vi "CH_LM Getting Started.vi"(5 "ID Query? (T: Yes)":bool, 7 "Reset? (F: No)":bool) -> ()   [LabVIEW 2012, in "CH_LM.lvlib"]
doc: "This example VI can be used to test the communication with a connected LabMax device and a connected detector.\n\n<B>Hint:</B> The control on the rigt side are immediatly updated with values read from the device. So, if value does not change and no error occurred you request was executed sucessfully."
uses:
  CH_LM.lvlib
  <vilib>/Utility/error.llb/DialogType.ctl
  Instance           1 29Saved   CH_LM Getting Started .vi
  CH_LM Measurement Mode.ctl
  CH_LM Unit.ctl
  CH_LM Measurement Delivery Mode.ctl
  CH_LM Date Format.ctl
  CH_LM Meter Type.ctl
  CH_LM ProbeType.ctl
  CH_LM AnalogOutFullscaleVoltage.ctl
  CH_LM Numeric Resolution.ctl
  CH_LM Time.ctl
  CH_LM Statistics Display Item.ctl
  CH_LM Display Mode.ctl
  CH_LM Display Submode.ctl
  CH_LM View Mode.ctl
  CH_LM Trigger Bus Control.ctl
  CH_LM Trigger Source.ctl
  CH_LM Zoom Factor.ctl
  CH_LM File Information.ctl
  CH_LM Data Token.ctl
  CH_LM Streaming Data.ctl
  CH_LM System StatusCluster.ctl
  CH_LM ProbeQualifier.ctl
  CH_LM BaudRates.ctl
  CH_LM Parity.ctl
  CH_LM SerialConfiguration.ctl
panel:
  in  "stop":bool
  in  "Unlock? (True)":bool
  out "GUI Loop":i32
  out "stopping":bool
  out "SRQ error":bool
  out "SRQ":bool
  out "Polling error":bool
  out "Streaming error":bool
  out "Lock timed out":bool
  in  "Reset 4":bool
  out "Event error":errorcluster
  in  "Tab Control":T1(tab)
  out "Probe Diameter":dbl[unit] format="%#.2g"
  out "Probe Qualifier":T2
  in  "Update Probe":bool
  out "Responsitivity":dbl format="%#.1g"
  out "Calibration Date":timestamp format="%<%x>T"
  out "Serial Number":string
  out "Probe Type":T3
  out "Probe Model":string
  out "Meter Type":T4
  out "Serial Number":string
  out "Calibration Date":string
  out "Self-Test Result Message":string
  out "Self-Test Result Code":i32
  out "Lock timed out":bool
  out "Date":string
  out "Revision":string
  out "Instrument Driver Revision":string
  out "Vendor":string
  out "Module":string
  out "timed out?":bool
  in  "Address":i32=1
  in  "Serial Number":string
  in  "Serial Configuration\n(19200,N,8,1)":T5={"Baud Rate"=19200, "Parity"=0, "Data Bits"=8, "Stop Bits"=1} {"Parity" items=["None", "Odd", "Even"]; "Baud Rate" items=["9600"=9600, "19200"=19200, "38400"=38400, "57600"=57600, "115200"=115200]}
  in  "Pyroelectric Autoset":bool
  out "Zero Offset / W":dbl format="%#.3g"
  in  "Probe zero":bool
  in  "Reset":bool
  out "Number of files":i32
  out "Configuration Catalog":string[](array[string])
  in  "Delete":bool
  in  "Save":bool
  in  "Recall":bool
  in  "Rename":bool
  in  "Destination File Name (\"\")":string
  in  "Source File Name (\"\")":string
  in  "Update Catalog":bool
  in  "Range Option (Value)":enum16{"MINIMUM", "Value", "MAXIMUM"}(ring)=enum."Value"
  in  "Range":dbl=1.0
  in  "Auto Range (disable)":bool
  in  "Analog Out Fullscale Voltage (2V)":T8=enum."2 V"
  in  "Time / s (0:Auto)":i32
  in  "Number of Pulses (0:Auto)":i32
  in  "Aperture / cm² (1.0)":dbl=1.0 format="%#.2g"
  in  "Area Correction (disable)":bool
  in  "Compensation Factor (1.0)":dbl=1.0 format="%#.3g"
  in  "Gain Compensation (disable)":bool
  in  "Resolution (3 1/2)":T9
  in  "Speedup Status":T10
  in  "set Measurement Mode":bool
  in  "Unit":T11
  in  "Mode":T12
  in  "State (On)":bool=TRUE
  in  "Battery Auto Off Timer (1 min)":i32=1
  in  "Battery Auto Off (On)":bool
  in  "AC Auto Off Timer (1 min)":i32=1
  in  "AC Auto Off (On)":bool
  in  "Date Format (MDY)":T13
  in  "Time Stamp":timestamp format="%<%X\n%x>T"
  in  "Factor (1)":T14=enum."1"
  in  "Direction (horizontal)":bool
  in  "Display Mode":bool
  in  "Tune Clear":bool
  in  "Clear (false)":bool
  in  "Text (empty)":string
  in  "Contrast (0.5)":dbl=0.5 min=0.0 max=1.0 step=0.1 format="%#_3g"
  in  "Set Display Mode":bool
  in  "View Mode":T15
  in  "Display Submode":T16
  in  "Display Mode":T17
  in  "Sequence ID (0)":u32
  in  "Trigger Source":T18
  in  "Release":bool
  in  "Hold":bool
  in  "Trigger Bus Control (2)":T19=enum."Independent"
  in  "Trigger Delay (0µs)":dbl=5.0 format="%#.3g"
  in  "Trigger Slope (pos.)":bool=TRUE
  in  "Trigger Level (5%)":dbl=5.0 format="%#.3g"
  out "size":i32
  in  "set WL Table":bool
  in  "Wavelength Table":u32[](array[numeric])
  in  "WL correction (disable)":bool=TRUE
  in  "set Wavelength":bool
  in  "Option (Value)":enum16{"MINIMUM", "Value", "MAXIMUM"}(ring)=enum."Value"
  in  "Wavelength / nm":u32=123
  in  "Display Item List":T20[](array[typedef])=[enum."Mean"]
  in  "Sample Rate /Hz (10Hz)":dbl=10.0 format="%#.3e"
  in  "Sample Rate (1)":i32=1
  in  "Batch Time (00:01:00)":T21={"Hours"=0, "Minutes"=1, "Seconds"=0}
  in  "Batch Size (2)":i32=2
  in  "Number of Bins (7)":i32=7
  in  "Restart Mode (f:manual)":bool=TRUE
  in  "Polling active":bool
  out "Head Temperature":dbl[unit](slide)=273.15 scale=263.15..373.15
  in  "Intervall / ms":u32=500
  out "Status":T22
  out "Status Description":string
  in  "Reset 2":bool
  out "Polling error":errorcluster
  in  "send SCPI":bool
  out "Response":string
  in  "NofStrings (-1:all)":i32=-1
  in  "SCPI Command/Query":string
  out "Response Array":string[](array[string])
  in  "Wait for SRQ active":bool
  out "Data String":string
  out "System Status":u32 format="%.0x"
  out "Status":T23
  out "Description":string
  out "SRQ error":errorcluster
  in  "Streaming active":bool
  out "Unit":string
  in  "Reset 3":bool
  out "Stream error":errorcluster
  in  "Delivery Mode":T24
  out "Steaming Data Chart":cluster{"Value":sgl, u32}[](graph)
  in  "Batch (start)":bool
  in  "Header (disable)":bool
  in  "Data Tokens":T25[](array[typedef])=[enum."Raw data"]
  out "Steaming Data Cluster":T26 {"Flags" format="%.0b"; "Unit ID" format="%.0b"; "Quad Distance"."Y" format="%#.1f"; "Quad Distance"."X" format="%#.1f"; "Value" format="%#.7e"}
  in  "Start/Stop (start)":bool=TRUE
  in  "Cycle Time (00:01:00)":T21={"Hours"=0, "Minutes"=1, "Seconds"=0}
  in  "File Name (\"\")":string
  in  "Sample Rate /Hz (10Hz) 2":dbl=10.0 format="%#.3e"
  in  "Trend Time (00:01:00)":T21={"Hours"=0, "Minutes"=1, "Seconds"=0}
  in  "Sampling Rate (1)":i32=1
  in  "Trend Size (2)":i32=2
  in  "Trend Histogram Bins (7)":i32=7
  in  "Trend Zoom (1)":T14=enum."1"
  in  "Trend Cycle (start)":bool=TRUE
  out "Current working directoy":string
  in  "Root":enum16{"\\loc", "\\usb"}(ring)
  in  "Destination (empty path)":path
  in  "Download":bool
  in  "Load from File":bool
  in  "Store into File":bool
  out "Catalog size":i32
  in  "Change Directory":bool
  in  "Create Directory":bool
  in  "Copy File":bool
  in  "Destination Name (\"\")":string
  in  "Rename":bool
  in  "Type":bool
  out "File":T27
  in  "Catalog index":u32
  in  "Delete File":bool
  out "Catalog":T27[](array[typedef])
  out "Bytes available":i32
  out "Bytes in use":i32
  in  "Read Catalog":bool
  # "Bus"
  # "External"
  # "Internal"
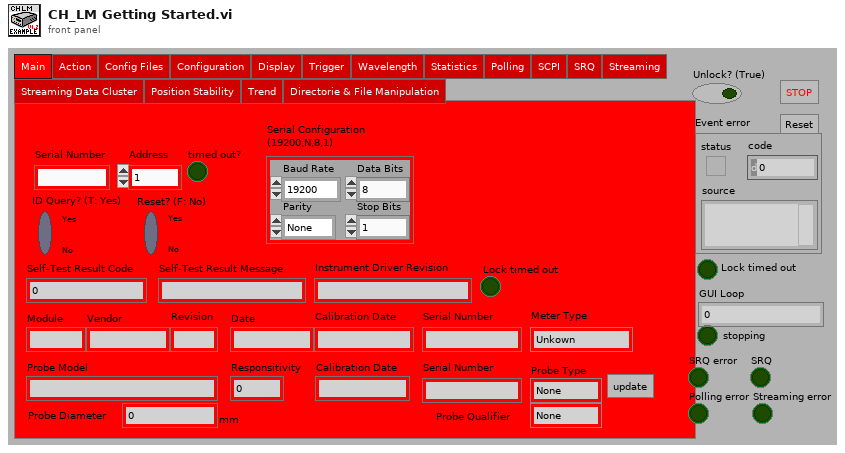
[diagram p1: front panel]
types:
  T1 = enum32{"Main", "Action", "Config Files", "Configuration", "Display", "Trigger", "Wavelength", "Statistics", "Polling", "SCPI", "SRQ", "Streaming", "Streaming Data Cluster", "Position Stability", "Trend", "Directorie & File Manipulation"}
  T2 = typedef "CH_LM.lvlib/CH_LM ProbeQualifier.ctl" = enum16{"None", "Single", "Quad", "No Spec"}
  T3 = typedef "CH_LM.lvlib/CH_LM ProbeType.ctl" = enum16{"None", "Thermopile", "Pyroelectric", "Optical"}
  T4 = typedef "CH_LM.lvlib/CH_LM Meter Type.ctl" = enum16{"Unkown", "TOP", "TO"}
  T5 = typedef "CH_LM.lvlib/CH_LM SerialConfiguration.ctl" = cluster{"Baud Rate":T6, "Parity":T7, "Data Bits":u16, "Stop Bits":u16}
  T6 = typedef "CH_LM.lvlib/CH_LM BaudRates.ctl" = u32
  T7 = typedef "CH_LM.lvlib/CH_LM Parity.ctl" = u16
  T8 = typedef "CH_LM.lvlib/CH_LM AnalogOutFullscaleVoltage.ctl" = enum16{"1 V", "2 V", "4 V"}
  T9 = typedef "CH_LM.lvlib/CH_LM Numeric Resolution.ctl" = enum16{"3½", "4½", "5½", "6½"}
  T10 = cluster{"Host":bool, "Analog":bool, "Numeric":bool, "Tune":bool}
  T11 = typedef "CH_LM.lvlib/CH_LM Unit.ctl" = enum16{"Joule", "Watt", "dBm"}
  T12 = typedef "CH_LM.lvlib/CH_LM Measurement Mode.ctl" = enum16{"Energy", "Power"}
  T13 = typedef "CH_LM.lvlib/CH_LM Date Format.ctl" = enum16{"MDY", "DMY"}
  T14 = typedef "CH_LM.lvlib/CH_LM Zoom Factor.ctl" = enum16{"Auto", "1", "2", "5", "10", "20"}
  T15 = typedef "CH_LM.lvlib/CH_LM View Mode.ctl" = enum16{"Scroll", "Fit to Screen", "Strip Chart", "Bar Chart"}
  T16 = typedef "CH_LM.lvlib/CH_LM Display Submode.ctl" = enum16{"Numbers", "Histogram", "Chart"}
  T17 = typedef "CH_LM.lvlib/CH_LM Display Mode.ctl" = enum16{"Non-Statistics", "Statistics", "Position Stability", "Tune", "Trend"}
  T18 = typedef "CH_LM.lvlib/CH_LM Trigger Source.ctl" = enum16{"Internal", "External", "Bus"}
  T19 = typedef "CH_LM.lvlib/CH_LM Trigger Bus Control.ctl" = enum16{"Host", "Guest", "Independent"}
  T20 = typedef "CH_LM.lvlib/CH_LM Statistics Display Item.ctl" = enum16{"Mean", "Minimum", "Maximum", "Standard Deviation", "1 Sigma", "2 Sigma", "3 Sigma", "Range", "Dose", "Missed"}
  T21 = typedef "CH_LM.lvlib/CH_LM Time.ctl" = cluster{"Hours":i32, "Minutes":i32, "Seconds":i32}
  T22 = cluster{"Battery":bool, "Temp":bool, "Probe":bool, "Drive":bool, "Autoset":bool, "Batch":bool, "Trend":bool, "Power":bool, "Trigger":bool, "Flash":bool, "FIFO":bool}
  T23 = typedef "CH_LM.lvlib/CH_LM System StatusCluster.ctl" = cluster{"Battery":bool, "Temp":bool, "Probe":bool, "Drive":bool, "Autoset":bool, "Batch":bool, "Trend":bool, "Power":bool, "Trigger":bool, "Flash":bool, "FIFO":bool, "Remote":bool, "Copy":bool}
  T24 = typedef "CH_LM.lvlib/CH_LM Measurement Delivery Mode.ctl" = enum16{"Last", "Stream"}
  T25 = typedef "CH_LM.lvlib/CH_LM Data Token.ctl" = enum16{"Raw data", "Quad distance", "Formated data", "Unit", "Pulse period", "Flags", "Sequence ID"}
  T26 = typedef "CH_LM.lvlib/CH_LM Streaming Data.ctl" = cluster{"Value":sgl, "Quad Distance":cluster{"X":sgl, "Y":sgl}, "Display Data":cluster{"Format ID":u8, "Scale ID":u8}, "Unit ID":u8, "Flags":u32, "Pulse Period":u32, "Sequence ID":u32, "Unit String":string}
  T27 = typedef "CH_LM.lvlib/CH_LM File Information.ctl" = cluster{"File name":string, "File type":string, "File size":i32}
  T28 = typedef "CH_LM.lvlib/CH_LM System Status.ctl" = u32
  T29 = cluster{"[0]":bool, "[1]":bool, "[2]":bool, "[3]":bool}
  T30 = cluster{"[0]":bool, "[1]":bool, "[2]":bool, "[3]":bool, "[4]":bool, "[5]":bool, "[6]":bool, "[7]":bool, "[8]":bool, "[9]":bool, "[10]":bool}
  T31 = typedef "DialogType.ctl" = u16
  T32 = typedef "CH_LM.lvlib/CH_LM Communication Mode.ctl" = enum16{"None", "USB", "GPIB", "RS232"}
  T33 = typedef "CH_LM File Information.ctl" = cluster{"File name":string, "File type":string, "File size":i32}
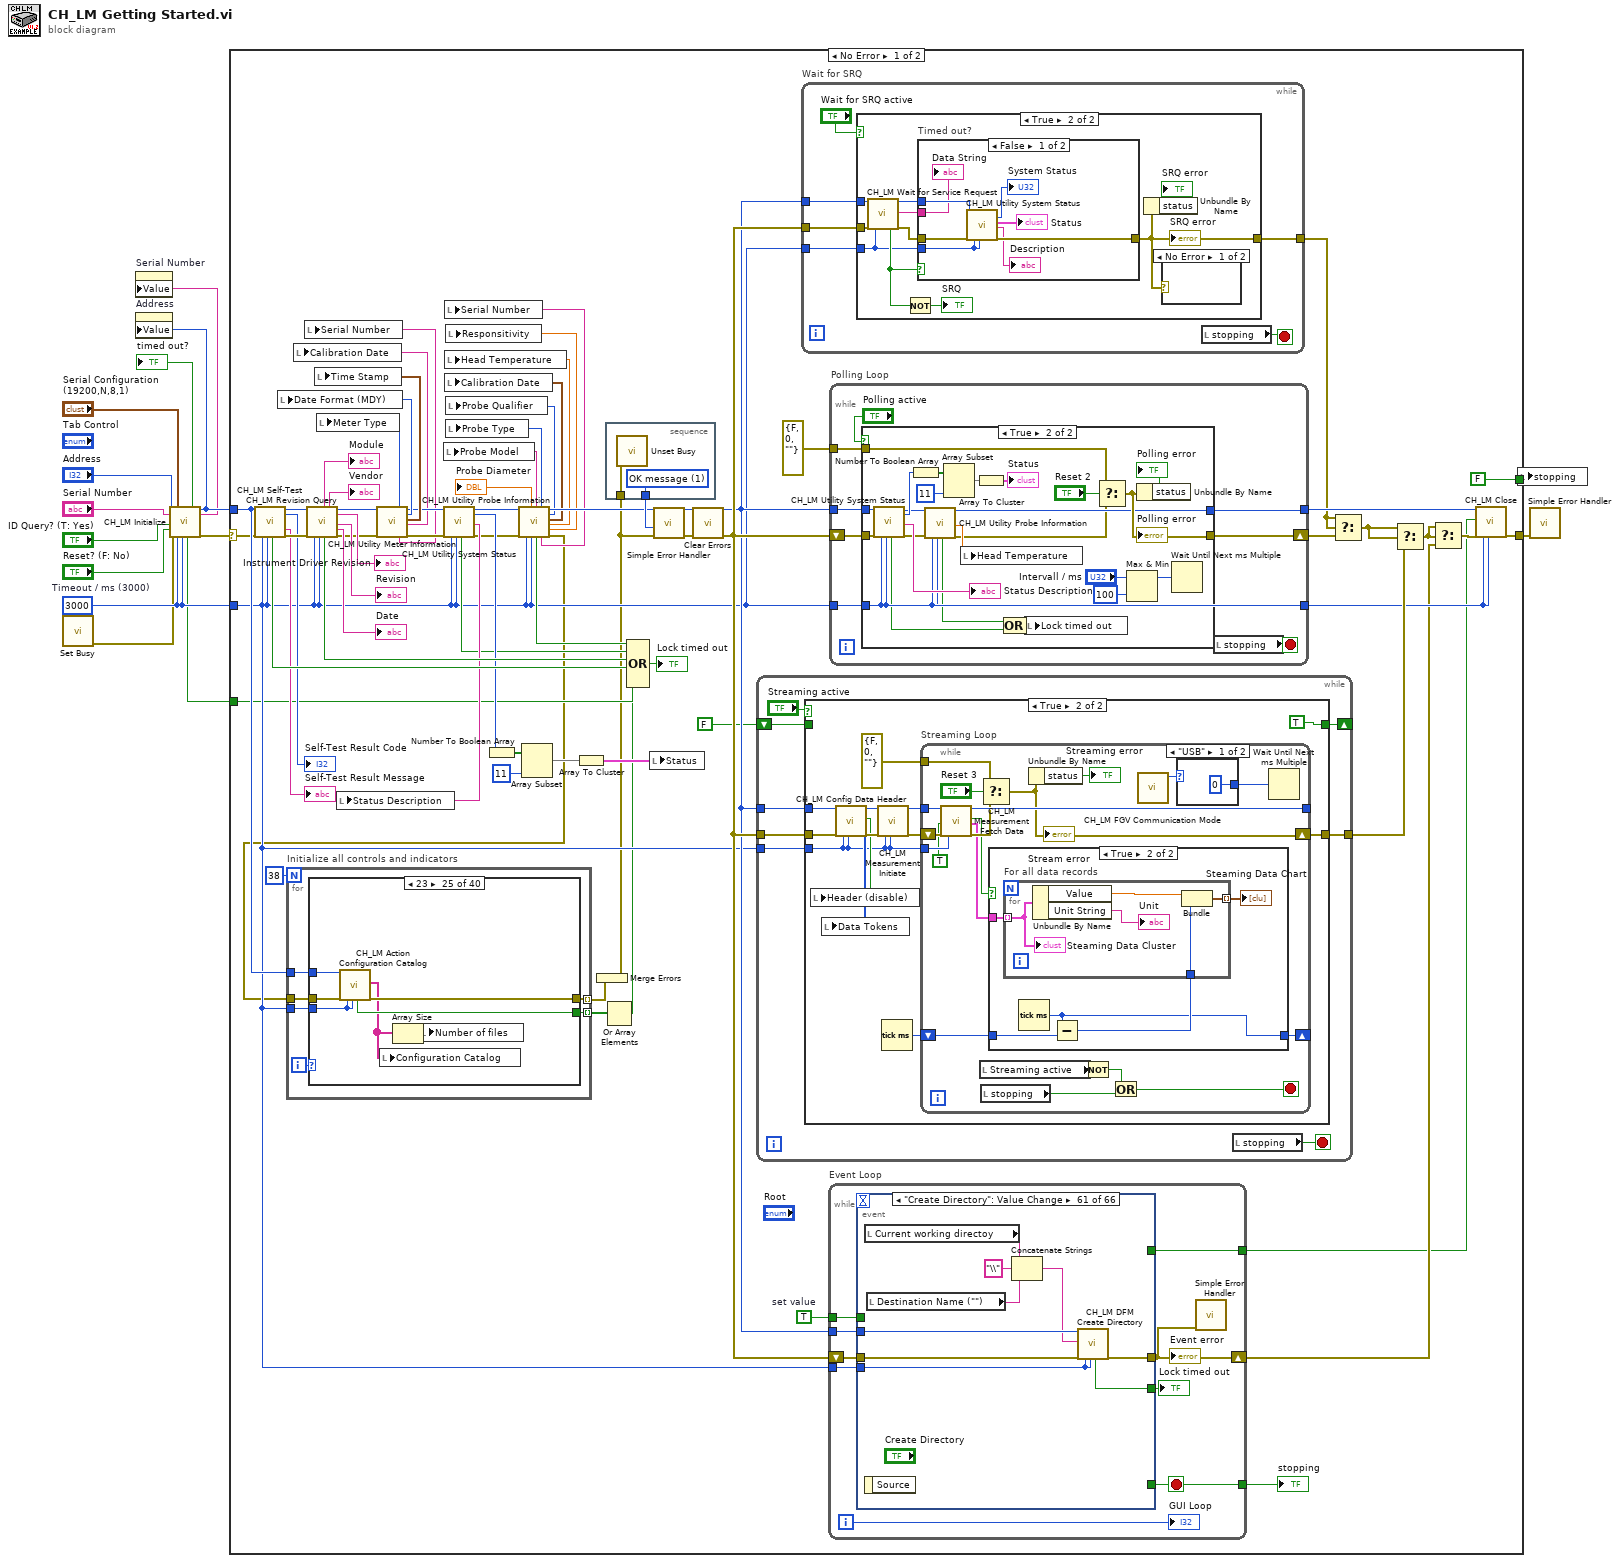
[diagram p0: block diagram]
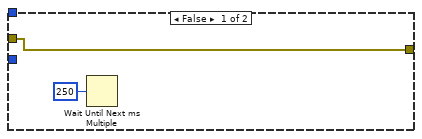
[diagram p2: hidden frame]
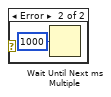
[diagram p3: hidden frame]
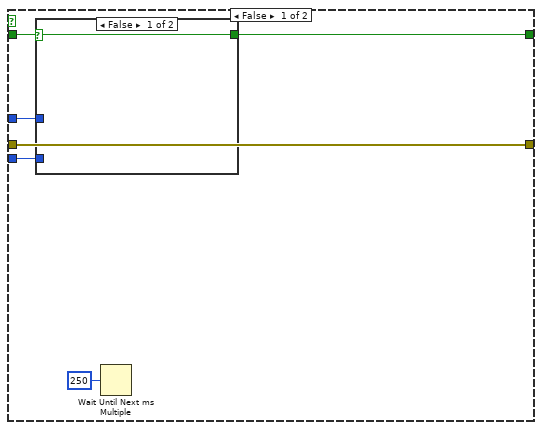
[diagram p5: hidden frame]
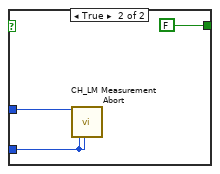
[diagram p6: hidden frame]
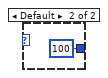
[diagram p7: hidden frame]
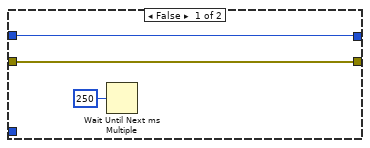
[diagram p9: hidden frame]
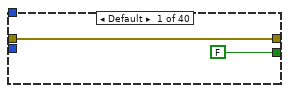
[diagram p10: hidden frame]
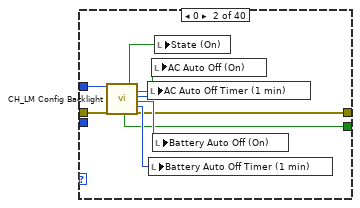
[diagram p11: hidden frame]
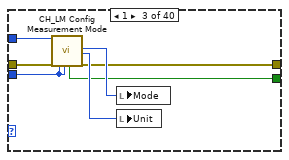
[diagram p12: hidden frame]
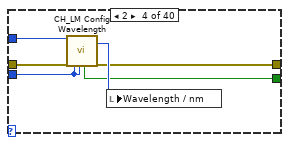
[diagram p13: hidden frame]
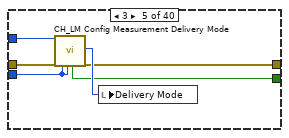
[diagram p14: hidden frame]
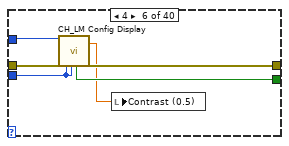
[diagram p15: hidden frame]
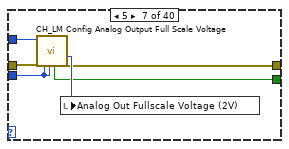
[diagram p16: hidden frame]
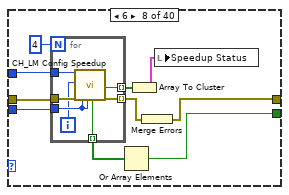
[diagram p17: hidden frame]
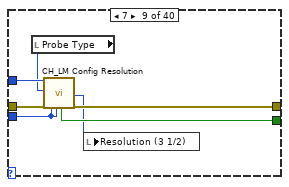
[diagram p18: hidden frame]
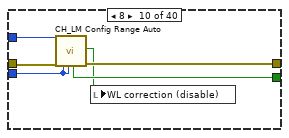
[diagram p19: hidden frame]
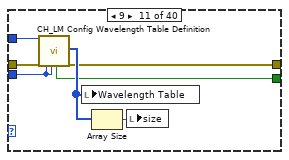
[diagram p20: hidden frame]
diagram:
  w11 = 3000  # Timeout / ms (3000)
  n1 = call <vilib>:"Set Busy.vi"() -> ("error out"=w4:errorcluster)  [unwired: 4 in, 7 out]
  n2 = call "CH_LM Initialize.vi"("Address"="Address", "Serial Number"="Serial Number", "ID Query (True)"="ID Query? (T: Yes)", "Reset (False)"="Reset? (F: No)", "error in (no error)"=w4, "Serial Configuration\n(19200,N,8,1)"="Serial Configuration\n(19200,N,8,1)", "Timeout / ms (3000)"=w11, "Lock Timeout / ms (1000)"=w11) -> ("Lock timed out"=w10:bool, "timed out?"=→"timed out?":bool, "Meter Index"=w3:i32, "Serial Number"=w2:string, "error out"=w8:errorcluster)  [unwired: 7 out]
  n3 = property on="Serial Number" class="Str"("Value"=w2) -> ()  [unwired: 2 in, 2 out]
  n4 = property on="Address" class="DigNum (strict)"("Value"=w3) -> ()  [unwired: 2 in, 2 out]
  n5 = case shown="No Error" w8 {
    selector: w8 -> [w28 w1239]
    tunnel: [w83 w1239] -> w14
    tunnel: w3 -> [w29 _]
    tunnel: w11 -> [w27 _]
    tunnel: w10 -> [w25 _]
    tunnel: [FALSE _] -> w7
    frame No Error {
      w64 = TRUE  # set value
      n6 = call "CH_LM Self-Test.vi"("Meter Index"=w29, "error in (no error)"=w28, "Timeout / ms (3000)"=w27, "Lock Timeout / ms (1000)"=w27) -> ("Lock timed out"=w70:bool, "Meter Index"=w74:i32, "Self-Test Result Code"=→"Self-Test Result Code":i32, "Self-Test Result Message"=→"Self-Test Result Message":string, "error out"=w73:errorcluster)  [unwired: 11 out]
      n7 = call "CH_LM Revision Query.vi"("Meter Index"=w74, "error in (no error)"=w73, "Timeout / ms (3000)"=w27, "Lock Timeout / ms (1000)"=w27) -> ("Module"=→"Module":string, "Lock timed out"=w71:bool, "Vendor"=→"Vendor":string, "Meter Index"=w47:i32, "Instrument Driver Revision"=→"Instrument Driver Revision":string, "Instrument Firmware Revision"=→"Revision":string, "Instrument Firmware Date"=→"Date":string, "error out"=w46:errorcluster)  [unwired: 8 out]
      n8 = call "CH_LM Utility Meter Information.vi"("Meter Index"=w47, "error in (no error)"=w46) -> ("Meter Type"=w44:T4, "Serial Number"=w42:string, "Meter Index"=w48:i32, "Date Format"=w51:T13, "Time Stamp"=w50:timestamp, "Calibration Date"=w43:string, "error out"=w45:errorcluster)  [unwired: 3 in, 8 out]
      n9 = local write "Date Format (MDY)"(w51) -> ()
      n10 = local write "Calibration Date"(w43) -> ()
      n11 = local write "Serial Number"(w42) -> ()
      n12 = local write "Time Stamp"(w50) -> ()
      n13 = local write "Meter Type"(w44) -> ()
      n14 = call "CH_LM Utility System Status.vi"("Meter Index"=w48, "error in (no error)"=w45, "Timeout / ms (3000)"=w27, "Lock Timeout / ms (1000)"=w27) -> ("Lock timed out"=w49:bool, "Meter Index"=w36:i32, "System Status"=w54:T28, "Status Description"=w52:string, "error out"=w37:errorcluster)  [unwired: 11 out]
      n15 = local write "Status Description"(w52) -> ()
      n16 = Number To Boolean Array(number=w54) -> (Boolean array=w56:bool[])
      n17 = call "CH_LM Utility Probe Information.vi"("Meter Index"=w36, "error in (no error)"=w37, "Timeout / ms (3000)"=w27, "Lock Timeout / ms (1000)"=w27) -> ("Probe Diameter"=→"Probe Diameter":dbl[unit], "Model"=w33:string, "Lock timed out"=w35:bool, "Probe Type"=w19:T3, "Serial Number"=w30:string, "Meter Index"=w34:i32, "Probe Qualifier"=w16:T2, "Calibration Date"=w32:timestamp, "Head Temperature"=w31:dbl[unit], "Responsitivity"=w17:dbl, "error out"=w22:errorcluster)  [unwired: 5 out]
      n18 = for "Initialize all controls and indicators" {
        N: 38 -> [_]
        tunnel: w29 -> [w217]
        tunnel: w22 -> [w213]
        tunnel: [w216] -> w23 mode=indexing
        tunnel: [w215] -> w26 mode=indexing
        tunnel: w27 -> [w214]
        i -> [w218]
        n19 = case shown="23" w218 {
          tunnel: w217 -> [_ w224 w234 w241 w247 w254 w259 w264 w284 w290 w296 w302 w308 w315 w321 w327 w332 w338 w344 w350 w356 w364 w370 w376 w386 w391 w397 w403 w409 w416 w422 w429 w437 w443 w449 w455 w462 w470 w480 w486]
          tunnel: w213 -> [w220 w223 w233 w240 w246 w253 w258 w266 w283 w289 w295 w301 w306 w314 w320 w326 w331 w337 w343 w349 w355 w363 w369 w375 w385 w389 w396 w402 w408 w415 w421 w428 w436 w442 w448 w454 w461 w469 w481 w485]
          tunnel: [w220 w222 w232 w237 w243 w250 w255 w263 w280 w286 w292 w298 w305 w311 w318 w323 w328 w334 w340 w347 w353 w360 w366 w372 w382 w388 w393 w399 w405 w412 w418 w425 w433 w440 w445 w451 w458 w466 w477 w482] -> w216
          tunnel: [FALSE ("Lock timed out") w221 w231 w238 w244 w251 w256 w267 w281 w287 w293 w299 w304 w312 w317 w324 w329 w335 w341 w346 w352 w361 w367 w373 w383 w387 w394 w400 w406 w413 w419 w426 w434 w439 w446 w452 w459 w467 w478 w483] -> w215
          tunnel: w214 -> [_ _ w230 w239 w245 w252 w257 w265 w282 w288 w294 w300 w307 w313 w319 w325 w330 w336 w342 w348 w354 w362 w368 w374 w384 w390 w395 w401 w407 w414 w420 w427 w435 w441 w447 w453 w460 w468 w479 w484]
          frame Default {
          }
          frame 0 {
            n20 = call "CH_LM Config Backlight.vi"("Meter Index"=w224, "error in (no error)"=w223) -> ("Lock timed out"=w221:bool, "State"=w225:bool, "AC Auto Off"=w226:bool, "AC Auto Off Timer / min"=w227:i32, "Battery Auto Off"=w228:bool, "Battery Auto Off Timer / min"=w229:i32, "error out"=w222:errorcluster)  [unwired: 6 in, 5 out]
            n21 = local write "AC Auto Off Timer (1 min)"(w227) -> ()
            n22 = local write "Battery Auto Off Timer (1 min)"(w229) -> ()
            n23 = local write "AC Auto Off (On)"(w226) -> ()
            n24 = local write "Battery Auto Off (On)"(w228) -> ()
            n25 = local write "State (On)"(w225) -> ()
          }
          frame 1 {
            n26 = call "CH_LM Config Measurement Mode.vi"("Meter Index"=w234, "error in (no error)"=w233, "Timeout / ms (3000)"=w230, "Lock Timeout / ms (1000)"=w230) -> ("Lock timed out"=w231:bool, "Mode"=w235:T12, "Unit"=w236:T11, "error out"=w232:errorcluster)  [unwired: 3 in, 9 out]
            n27 = local write "Mode"(w235) -> ()
            n28 = local write "Unit"(w236) -> ()
          }
          frame 2 {
            n29 = call "CH_LM Config Wavelength.vi"("Meter Index"=w241, "error in (no error)"=w240, "Timeout / ms (3000)"=w239, "Lock Timeout / ms (1000)"=w239) -> ("Lock timed out"=w238:bool, "Wavelength / nm"=w242:u32, "error out"=w237:errorcluster)  [unwired: 3 in, 10 out]
            n30 = local write "Wavelength / nm"(w242) -> ()
          }
          frame 3 {
            n31 = call "CH_LM Config Measurement Delivery Mode.vi"("Meter Index"=w247, "error in (no error)"=w246, "Timeout / ms (3000)"=w245, "Lock Timeout / ms (1000)"=w245) -> ("Lock timed out"=w244:bool, "Delivery Mode"=w248:T24, "error out"=w243:errorcluster)  [unwired: 2 in, 11 out]
            n32 = local write "Delivery Mode"(w248) -> ()
          }
          frame 4 {
            n33 = call "CH_LM Config Display.vi"("Meter Index"=w254, "error in (no error)"=w253, "Timeout / ms (3000)"=w252, "Lock Timeout / ms (1000)"=w252) -> ("Lock timed out"=w251:bool, "Contrast"=w249:dbl, "error out"=w250:errorcluster)  [unwired: 4 in, 9 out]
            n34 = local write "Contrast (0.5)"(w249) -> ()
          }
          frame 5 {
            n35 = call "CH_LM Config Analog Output Full Scale Voltage.vi"("Meter Index"=w259, "error in (no error)"=w258, "Timeout / ms (3000)"=w257, "Lock Timeout / ms (1000)"=w257) -> ("Lock timed out"=w256:bool, "Analog Out \nFullscale Voltage"=w260:T8, "error out"=w255:errorcluster)  [unwired: 2 in, 11 out]
            n36 = local write "Analog Out Fullscale Voltage (2V)"(w260) -> ()
          }
          frame 6 {
            n37 = for {
              N: 4 -> [_]
              tunnel: w264 -> [w277]
              tunnel: w265 -> [w275]
              tunnel: [w272] -> w268 mode=indexing
              tunnel: [w271] -> w269 mode=indexing
              tunnel: w266 -> [w276]
              tunnel: [w273] -> w262 mode=indexing
              i -> [w274]
              n38 = call "CH_LM Config Speedup.vi"("Meter Index"=w277, "Speedup Mode (0)"=w274, "error in (no error)"=w276, "Timeout / ms (3000)"=w275, "Lock Timeout / ms (1000)"=w275) -> ("Lock timed out"=w272:bool, "Status"=w271:bool, "error out"=w273:errorcluster)  [unwired: 2 in, 10 out]
            }
            n39 = Or Array Elements(Boolean array=w268) -> (logical OR=w267:bool)
            n40 = Array To Cluster(array=w269) -> (cluster=w270:T29)
            n41 = Merge Errors(w262) -> (w263:errorcluster)
            n42 = local write "Speedup Status"(w270) -> ()
          }
          frame 7 {
            n43 = local read "Probe Type"() -> (w278:T3)
            n44 = call "CH_LM Config Resolution.vi"("Meter Index"=w284, "Probe Type"=w278, "error in (no error)"=w283, "Timeout / ms (3000)"=w282, "Lock Timeout / ms (1000)"=w282) -> ("Lock timed out"=w281:bool, "Resolution (3 1/2)"=w279:T9, "error out"=w280:errorcluster)  [unwired: 2 in, 10 out]
            n45 = local write "Resolution (3 1/2)"(w279) -> ()
          }
          frame 8 {
            n46 = call "CH_LM Config Range Auto.vi"("Meter Index"=w290, "error in (no error)"=w289, "Timeout / ms (3000)"=w288, "Lock Timeout / ms (1000)"=w288) -> ("Lock timed out"=w287:bool, "Auto Range"=w285:bool, "error out"=w286:errorcluster)  [unwired: 2 in, 11 out]
            n47 = local write "WL correction (disable)"(w285) -> ()
          }
          frame 9 {
            n48 = call "CH_LM Config Wavelength Table Definition.vi"("Meter Index"=w296, "error in (no error)"=w295, "Timeout / ms (3000)"=w294, "Lock Timeout / ms (1000)"=w294) -> ("Lock timed out"=w293:bool, "Wavelength Table"=w297:u32[], "error out"=w292:errorcluster)  [unwired: 3 in, 10 out]
            n49 = local write "Wavelength Table"(w297) -> ()
            n50 = Array Size(array=w297) -> (size(s)=w291:i32)
            n51 = local write "size"(w291) -> ()
          }
          frame 10 {
            n52 = call "CH_LM Config Gain Compensation State.vi"("Meter Index"=w302, "error in (no error)"=w301, "Timeout / ms (3000)"=w300, "Lock Timeout / ms (1000)"=w300) -> ("Lock timed out"=w299:bool, "Gain Compensation"=w303:bool, "error out"=w298:errorcluster)  [unwired: 2 in, 11 out]
            n53 = local write "Gain Compensation (disable)"(w303) -> ()
          }
          frame 11 {
            n54 = call "CH_LM Config Gain Compensation.vi"("Meter Index"=w308, "error in (no error)"=w306, "Timeout / ms (3000)"=w307, "Lock Timeout / ms (1000)"=w307) -> ("Lock timed out"=w304:bool, "Compensation Factor"=w309:dbl, "error out"=w305:errorcluster)  [unwired: 2 in, 11 out]
            n55 = local write "Compensation Factor (1.0)"(w309) -> ()
          }
          frame 12 {
            n56 = call "CH_LM Config Area Correction State.vi"("Meter Index"=w315, "error in (no error)"=w314, "Timeout / ms (3000)"=w313, "Lock Timeout / ms (1000)"=w313) -> ("Lock timed out"=w312:bool, "Area Correction"=w310:bool, "error out"=w311:errorcluster)  [unwired: 2 in, 11 out]
            n57 = local write "Area Correction (disable)"(w310) -> ()
          }
          frame 13 {
            n58 = call "CH_LM Config Aperture.vi"("Meter Index"=w321, "error in (no error)"=w320, "Timeout / ms (3000)"=w319, "Lock Timeout / ms (1000)"=w319) -> ("Lock timed out"=w317:bool, "Aperture / cm²"=w316:dbl, "error out"=w318:errorcluster)  [unwired: 2 in, 11 out]
            n59 = local write "Aperture / cm² (1.0)"(w316) -> ()
          }
          frame 14 {
            n60 = call "CH_LM Action Probe Zero.vi"("Meter Index"=w327, "error in (no error)"=w326, "Timeout / ms (3000)"=w325, "Lock Timeout / ms (1000)"=w325) -> ("Lock timed out"=w324:bool, "Zero Offset / W"=w322:dbl, "error out"=w323:errorcluster)  [unwired: 1 in, 12 out]
            n61 = local write "Zero Offset / W"(w322) -> ()
          }
          frame 15 {
            n62 = call "CH_LM Config Display Smoothing Size Pulse.vi"("Meter Index"=w332, "error in (no error)"=w331, "Timeout / ms (3000)"=w330, "Lock Timeout / ms (1000)"=w330) -> ("Lock timed out"=w329:bool, "Number of Pulses"=w333:i32, "error out"=w328:errorcluster)  [unwired: 2 in, 11 out]
            n63 = local write "Number of Pulses (0:Auto)"(w333) -> ()
          }
          frame 16 {
            n64 = call "CH_LM Config Display Smoothing Size Time.vi"("Meter Index"=w338, "error in (no error)"=w337, "Timeout / ms (3000)"=w336, "Lock Timeout / ms (1000)"=w336) -> ("Lock timed out"=w335:bool, "Time / s"=w339:i32, "error out"=w334:errorcluster)  [unwired: 3 in, 10 out]
            n65 = local write "Time / s (0:Auto)"(w339) -> ()
          }
          frame 17 {
            n66 = call "CH_LM Config Statistics Restart Mode.vi"("Meter Index"=w344, "error in (no error)"=w343, "Timeout / ms (3000)"=w342, "Lock Timeout / ms (1000)"=w342) -> ("Lock timed out"=w341:bool, "Restart Mode"=w345:bool, "error out"=w340:errorcluster)  [unwired: 2 in, 11 out]
            n67 = local write "Restart Mode (f:manual)"(w345) -> ()
          }
          frame 18 {
            n68 = call "CH_LM Config Statistics Histogram Bin Count.vi"("Meter Index"=w350, "error in (no error)"=w349, "Timeout / ms (3000)"=w348, "Lock Timeout / ms (1000)"=w348) -> ("Lock timed out"=w346:bool, "Number of Bins"=w351:i32, "error out"=w347:errorcluster)  [unwired: 2 in, 11 out]
            n69 = local write "Number of Bins (7)"(w351) -> ()
          }
          frame 19 {
            n70 = call "CH_LM Config Statistics Batch Size.vi"("Meter Index"=w356, "error in (no error)"=w355, "Timeout / ms (3000)"=w354, "Lock Timeout / ms (1000)"=w354) -> ("Lock timed out"=w352:bool, "Batch Size"=w357:i32, "Sample Rate"=w358:i32, "error out"=w353:errorcluster)  [unwired: 3 in, 9 out]
            n71 = local write "Sample Rate (1)"(w358) -> ()
            n72 = local write "Batch Size (2)"(w357) -> ()
          }
          frame 20 {
            n73 = call "CH_LM Config Statistics Batch Time.vi"("Meter Index"=w364, "error in (no error)"=w363, "Timeout / ms (3000)"=w362, "Lock Timeout / ms (1000)"=w362) -> ("Lock timed out"=w361:bool, "Batch Time"=w365:T21, "Sample Rate / Hz"=w359:dbl, "error out"=w360:errorcluster)  [unwired: 3 in, 9 out]
            n74 = local write "Sample Rate /Hz (10Hz)"(w359) -> ()
            n75 = local write "Batch Time (00:01:00)"(w365) -> ()
          }
          frame 21 {
            n76 = call "CH_LM Config Statistics Display Item.vi"("Meter Index"=w370, "error in (no error)"=w369, "Timeout / ms (3000)"=w368, "Lock Timeout / ms (1000)"=w368) -> ("Lock timed out"=w367:bool, "Display Item List"=w371:T20[], "error out"=w366:errorcluster)  [unwired: 2 in, 11 out]
            n77 = local write "Display Item List"(w371) -> ()
          }
          frame 22 {
            n78 = call "CH_LM Config Display Mode.vi"("Meter Index"=w376, "Display Mode"="Display Mode", "error in (no error)"=w375, "Timeout / ms (3000)"=w374, "Lock Timeout / ms (1000)"=w374) -> ("Lock timed out"=w373:bool, "Display Submode"=w378:T16, "View Mode"=w379:T15, "error out"=w372:errorcluster)  [unwired: 3 in, 8 out]
            n79 = local write "Display Submode"(w378) -> ()
            n80 = local write "View Mode"(w379) -> ()
          }
          frame 23 {
            n81 = call "CH_LM Action Configuration Catalog.vi"("Meter Index"=w386, "error in (no error)"=w385, "Timeout / ms (3000)"=w384, "Lock Timeout / ms (1000)"=w384) -> ("Lock timed out"=w383:bool, "Configuration Catalog"=w381:string[], "error out"=w382:errorcluster)  [unwired: 13 out]
            n82 = local write "Configuration Catalog"(w381) -> ()
            n83 = Array Size(array=w381) -> (size(s)=w380:i32)
            n84 = local write "Number of files"(w380) -> ()
          }
          frame 24 {
            n85 = call "CH_LM Config Position Stability Cycle Duration.vi"("Meter Index"=w391, "error in (no error)"=w389, "Timeout / ms (3000)"=w390, "Lock Timeout / ms (1000)"=w390) -> ("Lock timed out"=w387:bool, "Cycle Time"=w392:T21, "error out"=w388:errorcluster)  [unwired: 2 in, 11 out]
            n86 = local write "Cycle Time (00:01:00)"(w392) -> ()
          }
          frame 25 {
            n87 = call "CH_LM Config Trigger Source.vi"("Meter Index"=w397, "error in (no error)"=w396, "Timeout / ms (3000)"=w395, "Lock Timeout / ms (1000)"=w395) -> ("Lock timed out"=w394:bool, "Trigger Source"=w398:T18, "error out"=w393:errorcluster)  [unwired: 2 in, 11 out]
            n88 = local write "Trigger Source"(w398) -> ()
          }
          frame 26 {
            n89 = call "CH_LM Config Trigger Level.vi"("Meter Index"=w403, "error in (no error)"=w402, "Timeout / ms (3000)"=w401, "Lock Timeout / ms (1000)"=w401) -> ("Lock timed out"=w400:bool, "Trigger Level / %"=w404:dbl, "error out"=w399:errorcluster)  [unwired: 2 in, 11 out]
            n90 = local write "Trigger Level (5%)"(w404) -> ()
          }
          frame 27 {
            n91 = call "CH_LM Config Trigger External.vi"("Meter Index"=w409, "error in (no error)"=w408, "Timeout / ms (3000)"=w407, "Lock Timeout / ms (1000)"=w407) -> ("Lock timed out"=w406:bool, "Trigger Slope"=w410:bool, "Trigger Delay / µs"=w411:dbl, "error out"=w405:errorcluster)  [unwired: 3 in, 9 out]
            n92 = local write "Trigger Slope (pos.)"(w410) -> ()
            n93 = local write "Trigger Delay (0µs)"(w411) -> ()
          }
          frame 28 {
            n94 = call "CH_LM Config Trigger Bus Control.vi"("Meter Index"=w416, "error in (no error)"=w415, "Timeout / ms (3000)"=w414, "Lock Timeout / ms (1000)"=w414) -> ("Lock timed out"=w413:bool, "Trigger Bus Control"=w417:T19, "error out"=w412:errorcluster)  [unwired: 2 in, 11 out]
            n95 = local write "Trigger Bus Control (2)"(w417) -> ()
          }
          frame 29 {
            n96 = call "CH_LM Config Range Auto.vi"("Meter Index"=w422, "error in (no error)"=w421, "Timeout / ms (3000)"=w420, "Lock Timeout / ms (1000)"=w420) -> ("Lock timed out"=w419:bool, "Auto Range"=w423:bool, "error out"=w418:errorcluster)  [unwired: 2 in, 11 out]
            n97 = local write "Auto Range (disable)"(w423) -> ()
          }
          frame 30 {
            n98 = local read "Range Option (Value)"() -> (w424:enum16{"MINIMUM", "Value", "MAXIMUM"})
            n99 = call "CH_LM Config Range.vi"("Meter Index"=w429, "Option (Value)"=w424, "error in (no error)"=w428, "Timeout / ms (3000)"=w427, "Lock Timeout / ms (1000)"=w427) -> ("Lock timed out"=w426:bool, "Granted Full Scale Range"=w430:dbl, "error out"=w425:errorcluster)  [unwired: 2 in, 10 out]
            n100 = local write "Range"(w430) -> ()
          }
          frame 31 {
            n101 = local read "Direction (horizontal)"() -> (w432:bool)
            n102 = local read "Display Mode"() -> (w431:bool)
            n103 = call "CH_LM Config Tune Zoom.vi"("Meter Index"=w437, "Display Mode"=w431, "Direction (horizontal)"=w432, "error in (no error)"=w436, "Timeout / ms (3000)"=w435, "Lock Timeout / ms (1000)"=w435) -> ("Lock timed out"=w434:bool, "Zoom Mode"=w438:T14, "error out"=w433:errorcluster)  [unwired: 2 in, 9 out]
            n104 = local write "Factor (1)"(w438) -> ()
          }
          frame 32 {
            n105 = call "CH_LM Config Trend Zoom.vi"("Meter Index"=w443, "error in (no error)"=w442, "Timeout / ms (3000)"=w441, "Lock Timeout / ms (1000)"=w441) -> ("Lock timed out"=w439:bool, "Zoom Mode"=w444:T14, "error out"=w440:errorcluster)  [unwired: 2 in, 11 out]
            n106 = local write "Trend Zoom (1)"(w444) -> ()
          }
          frame 33 {
            n107 = call "CH_LM Config Trend Histogram Bin Count.vi"("Meter Index"=w449, "error in (no error)"=w448, "Timeout / ms (3000)"=w447, "Lock Timeout / ms (1000)"=w447) -> ("Lock timed out"=w446:bool, "Number of Bins"=w450:i32, "error out"=w445:errorcluster)  [unwired: 2 in, 11 out]
            n108 = local write "Trend Histogram Bins (7)"(w450) -> ()
          }
          frame 34 {
            n109 = call "CH_LM Config Trend Size.vi"("Meter Index"=w455, "error in (no error)"=w454, "Timeout / ms (3000)"=w453, "Lock Timeout / ms (1000)"=w453) -> ("Lock timed out"=w452:bool, "Trend Size"=w456:i32, "Sampling Rate"=w457:i32, "error out"=w451:errorcluster)  [unwired: 3 in, 9 out]
            n110 = local write "Sampling Rate (1)"(w457) -> ()
            n111 = local write "Trend Size (2)"(w456) -> ()
          }
          frame 35 {
            n112 = call "CH_LM Config Trend Time.vi"("Meter Index"=w462, "error in (no error)"=w461, "Timeout / ms (3000)"=w460, "Lock Timeout / ms (1000)"=w460) -> ("Lock timed out"=w459:bool, "Trend Time"=w463:T21, "Sample Rate / Hz"=w464:dbl, "error out"=w458:errorcluster)  [unwired: 3 in, 9 out]
            n113 = local write "Sample Rate /Hz (10Hz) 2"(w464) -> ()
            n114 = local write "Trend Time (00:01:00)"(w463) -> ()
          }
          frame 38 {
            n115 = call "CH_LM DFM Change Directory.vi"("Meter Index"=w470, "error in (no error)"=w469, "Timeout / ms (3000)"=w468, "Lock Timeout / ms (1000)"=w468) -> ("Lock timed out"=w467:bool, "Woring Directory"=w465:string, "error out"=w466:errorcluster)  [unwired: 2 in, 11 out]
            n116 = local write "Current working directoy"(w465) -> ()
          }
          frame 36 {
            w476 = u32 0 ("Catalog index")
            n117 = property on="Catalog index" class="DigNum (strict)"("Value"=w476) -> ()  [unwired: 2 in, 2 out]
            n118 = call "CH_LM DFM Catalog.vi"("Meter Index"=w480, "error in (no error)"=w481, "Timeout / ms (3000)"=w479, "Lock Timeout / ms (1000)"=w479) -> ("Lock timed out"=w478:bool, "Bytes in use"=w471:i32, "Bytes available"=w472:i32, "Catalog"=w473:T27[], "error out"=w477:errorcluster)  [unwired: 11 out]
            n119 = local write "Bytes in use"(w471) -> ()
            n120 = local write "Bytes available"(w472) -> ()
            n121 = local write "Catalog"(w473) -> ()
            n122 = Index Array(array=w473, index=w476) -> (element=w475:T27)
            n123 = Array Size(array=w473) -> (size(s)=w474:i32)
            n124 = local write "Catalog size"(w474) -> ()
            n125 = local write "File"(w475) -> ()
          }
          frame 37 {
            n126 = call "CH_LM Config Data Header.vi"("Meter Index"=w486, "error in (no error)"=w485, "Timeout / ms (3000)"=w484, "Lock Timeout / ms (1000)"=w484) -> ("Lock timed out"=w483:bool, "Data Header"=w487:bool, "Data Tokens"=w488:T25[], "error out"=w482:errorcluster)  [unwired: 3 in, 9 out]
            n127 = local write "Header (disable)"(w487) -> ()
            n128 = local write "Data Tokens"(w488) -> ()
          }
        }
      }
      n129 = local write "Probe Model"(w33) -> ()
      n130 = local write "Serial Number"(w30) -> ()
      n131 = local write "Head Temperature"(w31) -> ()
      n132 = local write "Calibration Date"(w32) -> ()
      n133 = local write "Responsitivity"(w17) -> ()
      n134 = local write "Probe Qualifier"(w16) -> ()
      n135 = local write "Probe Type"(w19) -> ()
      n136 = Array Subset(array=w56, length=11) -> (w57:bool[])  [unwired: 1 in]
      n137 = Array To Cluster(array=w57) -> (cluster=w53:T30)
      n138 = Merge Errors(w23) -> (w20:errorcluster)
      n139 = Or Array Elements(Boolean array=w26) -> (logical OR=w24:bool)
      n140 = stacked-sequence {
        tunnel: [w212] -> w41
        tunnel: w20 -> [w211]
        frame #0 {
          w212 = T31 1 items=["no dialog", "OK message", "continue or stop message", "OK message + warnings", "continue/stop + warnings"] ("type of dialog (OK msg:1)")
          n141 = call <vilib>:"Unset Busy.vi"("error in (no error)"=w211) -> ()  [unwired: 1 in, 10 out]
        }
      }
      n142 = Compound Arithmetic op=OR(w35, w49, w71, w70, w25, w24) -> (→"Lock timed out":bool)
      n143 = local write "Status"(w53) -> ()
      n144 = call <vilib>:"Simple Error Handler.vi"("type of dialog (OK msg:1)"=w41, "error in (no error)"=w20) -> ("error out"=w40:errorcluster)  [unwired: 7 out]
      n145 = call <vilib>:"Clear Errors.vi"("error in (no error)"=w40) -> ("error out"=w39:errorcluster)  [unwired: 1 in, 5 out]
      n146 = while {
        tunnel: [w119] -> w81
        tunnel: w39 -> [w117]
        tunnel: w34 -> [w116]
        tunnel: w27 -> [w115]
        shift-right: [w113] -> _
        shift-left: FALSE -> [w112]
        stop <- w114 stop-if-true
        n147 = case shown="True" "Streaming active" {
          tunnel: [w124 w131] -> w119
          tunnel: w115 -> [w120 w132]
          tunnel: w116 -> [w122 w135]
          tunnel: w117 -> [w124 w134]
          tunnel: [w121 TRUE] -> w113
          tunnel: w112 -> [w123 _]
          frame False {
            n148 = case shown="False" w123 {
              selector: w123 -> [w126 _]
              tunnel: w122 -> [_ w129]
              tunnel: [w126 FALSE] -> w121
              tunnel: w120 -> [_ w127]
              frame False {
              }
              frame True {
                n149 = call "CH_LM Measurement Abort.vi"("Meter Index"=w129, "Timeout / ms (3000)"=w127, "Lock Timeout / ms (1000)"=w127) -> ()  [unwired: 1 in, 16 out]
              }
            }
            n150 = Wait Until Next ms Multiple(millisecond multiple=u32 250) -> ()  [unwired: 1 out]
          }
          frame True {
            n151 = call "CH_LM Config Data Header.vi"("Meter Index"=w135, "error in (no error)"=w134, "Timeout / ms (3000)"=w132, "Lock Timeout / ms (1000)"=w132) -> ("Meter Index"=w139:i32, "Data Header"=w137:bool, "Data Tokens"=w136:T25[], "error out"=w138:errorcluster)  [unwired: 3 in, 9 out]
            n152 = local write "Header (disable)"(w137) -> ()
            n153 = local write "Data Tokens"(w136) -> ()
            n154 = call "CH_LM Measurement Initiate.vi"("Meter Index"=w139, "error in (no error)"=w138, "Timeout / ms (3000)"=w132, "Lock Timeout / ms (1000)"=w132) -> ("Meter Index"=w142:i32, "error out"=w141:errorcluster)  [unwired: 14 out]
            n155 = Tick Count (ms)() -> (millisecond timer value=w133:u32)
            n156 = while "Streaming Loop" {
              tunnel: w142 -> [w162]
              shift-right: [w150] -> w131
              shift-left: w141 -> [w161]
              tunnel: [w160] -> _
              tunnel: w132 -> [w159]
              tunnel: errorcluster {"status"=FALSE, "code"=0, "source"=""} ("error in (no error)") -> [w157]
              shift-right: [w152] -> _
              shift-left: w133 -> [w153]
              stop <- w143 stop-if-true
              n157 = call "CH_LM Measurement Fetch Data.vi"("Meter Index"=w162, "All Records? (F)"=TRUE, "error in (no error)"=w161, "Timeout / ms (1000)"=w159) -> ("Meter Index"=w160:i32, "Data OK"=w155:bool, "Data Array"=w154:T26[], "error out"=w156:errorcluster)  [unwired: 1 in, 11 out]
              n158 = local read "Streaming active"() -> (w146:bool)
              n159 = Select(t=w157, s="Reset 3", f=w156) -> (s? t:f=w150:errorcluster)
              "Stream error" <- w150
              n160 = local read "stopping"() -> (w144:bool)
              n161 = case shown="True" w155 {
                tunnel: w154 -> [_ w170]
                tunnel: w153 -> [w165 w168]
                tunnel: [w165 w166] -> w152
                frame False {
                }
                frame True {
                  n162 = Tick Count (ms)() -> (millisecond timer value=w166:u32)
                  n163 = Subtract(x=w166, y=w168) -> (x-y=w167:u32)
                  n164 = for "For all data records" {
                    tunnel: w170 -> [w175] mode=indexing
                    tunnel: [w173] -> w169 mode=indexing
                    tunnel: w167 -> [w172]
                    n165 = Unbundle By Name(w175) -> ("Value"=w174:sgl, "Unit String"=→"Unit":string)
                    n166 = Bundle("Value"=w174, w172) -> (w173:cluster{"Value":sgl, u32})  [unwired: 1 out]
                    "Steaming Data Cluster" <- w175
                  }
                  "Steaming Data Chart" <- w169
                }
              }
              n167 = Unbundle By Name(w150) -> ("status"=→"Streaming error":bool)
              n168 = Not(x=w146) -> (.not. x?=w145:bool)
              n169 = Or(x=w145, y=w144) -> (x .or. y?=w143:bool)
              n170 = call "CH_LM FGV Communication Mode.vi"() -> ("Communication Mode"=w148:T32)  [unwired: 3 in, 5 out]
              n171 = case shown="\"USB\"" w148 {
                tunnel: [u32 0 ("millisecond multiple") u32 100 ("millisecond multiple")] -> w149
                frame "USB" {
                }
                frame Default {
                }
              }
              n172 = Wait Until Next ms Multiple(millisecond multiple=w149) -> ()  [unwired: 1 out]
            }
          }
        }
        n173 = local read "stopping"() -> (w114:bool)
      }
      n174 = while "Wait for SRQ" {
        tunnel: w27 -> [w85]
        tunnel: w39 -> [w88]
        tunnel: w34 -> [w87]
        tunnel: [w86] -> w63
        stop <- w89 stop-if-true
        n175 = case shown="True" "Wait for SRQ active" {
          tunnel: w88 -> [w91 w101]
          tunnel: w87 -> [_ w100]
          tunnel: [w91 w94] -> w86
          tunnel: w85 -> [_ w92]
          frame False {
            n176 = Wait Until Next ms Multiple(millisecond multiple=u32 250) -> ()  [unwired: 1 out]
          }
          frame True {
            n177 = call "CH_LM Wait for Service Request.vi"("Meter Index"=w100, "error in (no error)"=w101, "Timeout / ms (1000)"=w92) -> ("timed out?"=w97:bool, "Meter Index"=w93:i32, "Data String"=w99:string, "error out"=w98:errorcluster)  [unwired: 13 out]
            n178 = Not(x=w97) -> (.not. x?=→"SRQ":bool)
            n179 = case "Timed out?" shown="False" w97 {
              tunnel: w99 -> [w105 _]
              tunnel: w98 -> [w110 w111]
              tunnel: [w109 w111] -> w94
              tunnel: w93 -> [w108 _]
              tunnel: w92 -> [w107 _]
              frame False {
                n180 = call "CH_LM Utility System Status.vi"("Meter Index"=w108, "error in (no error)"=w110, "Timeout / ms (3000)"=w107, "Lock Timeout / ms (1000)"=w107) -> ("System Status"=→"System Status":T28, "Status"=→"Status":T23, "Status Description"=→"Description":string, "error out"=w109:errorcluster)  [unwired: 12 out]
                "Data String" <- w105
              }
              frame True {
              }
            }
            "SRQ error" <- w94
            n181 = Unbundle By Name(w94) -> ("status"=→"SRQ error":bool)
            n182 = case shown="No Error" w94 {
              frame No Error {
              }
              frame Error {
                n183 = Wait Until Next ms Multiple(millisecond multiple=u32 1000) -> ()  [unwired: 1 out]
              }
            }
          }
        }
        n184 = local read "stopping"() -> (w89:bool)
      }
      n185 = while "Event Loop" {
        tunnel: [w497] -> w65
        tunnel: w34 -> [w496]
        tunnel: w27 -> [w494]
        shift-right: [w492] -> w58
        shift-left: w39 -> [w495]
        tunnel: w64 -> [w491]
        tunnel: [w489] -> w38
        i -> [w490]
        stop <- w497 stop-if-true
        n186 = event shown="[60] \"Create Directory\": Value Change" {
          selector: _ -> [_ _ _ _ _ _ _ _ _ _ _ _ _ _ _ _ _ _ _ _ _ _ _ _ _ _ _ _ _ _ _ _ _ _ _ _ _ _ _ _ _ _ _ _ _ _ _ _ _ _ _ _ _ _ _ _ _ _ _ _ _ _ _ _ _ _]
          dyn-events: _ -> [_ _ _ _ _ _ _ _ _ _ _ _ _ _ _ _ _ _ _ _ _ _ _ _ _ _ _ _ _ _ _ _ _ _ _ _ _ _ _ _ _ _ _ _ _ _ _ _ _ _ _ _ _ _ _ _ _ _ _ _ _ _ _ _ _ _]
          timeout: _ -> [_ _ _ _ _ _ _ _ _ _ _ _ _ _ _ _ _ _ _ _ _ _ _ _ _ _ _ _ _ _ _ _ _ _ _ _ _ _ _ _ _ _ _ _ _ _ _ _ _ _ _ _ _ _ _ _ _ _ _ _ _ _ _ _ _ _]
          tunnel: [_ w501 _ _ _ _ _ _ _ _ _ _ _ _ _ _ _ _ _ _ _ _ _ _ _ _ _ _ _ _ _ _ _ _ _ _ _ _ _ _ _ _ _ _ _ _ _ _ _ _ _ _ _ _ _ _ _ _ _ _ _ _ _ _ _ _] -> w497
          tunnel: w496 -> [_ _ w506 w526 w540 w553 w564 w571 w583 w598 w603 w619 w635 w647 w663 w693 w705 w718 w730 w742 w753 w765 w776 w788 w800 w812 w824 w838 w852 w864 w879 w886 w892 w898 w905 w911 w923 w929 w941 w953 w967 w979 w984 w989 w995 w1000 w1010 w1023 w1028 w1042 w1049 w1061 w1073 w1087 w1101 w1112 w1125 _ w1142 w1153 w1167 w1180 w1187 w1199 w1215 w1238]
          tunnel: w495 -> [w498 w500 _ w525 w539 w552 w563 w570 w582 w597 w602 w618 w634 w646 w662 w692 w704 w717 w729 w741 w752 w764 w775 w787 w799 w811 w823 w837 w851 w863 w878 w885 w891 w897 w904 w910 w922 w928 w940 w952 w966 w978 w983 w988 w994 w999 w1009 w1022 w1027 w1041 w1048 w1060 w1072 w1086 w1100 w1111 w1124 w1132 w1141 w1150 w1166 w1179 w1186 w1198 w1214 w1237]
          tunnel: w494 -> [_ _ w503 w522 w534 w547 w556 w569 w581 w596 w601 w616 w626 w636 w661 w689 w699 w712 w724 w736 w747 w759 w771 w778 w793 w806 w818 w832 w846 w858 w872 w884 w890 w896 w903 w909 w917 w927 w932 w945 w958 w969 w982 w987 w991 w998 w1004 w1014 w1026 w1029 w1047 w1051 w1063 w1076 w1088 w1110 w1123 _ w1140 w1147 w1165 w1174 w1185 w1197 w1212 w1228]
          tunnel: [w498 w500 w504 w508 w530 w548 w554 w567 w579 w595 w599 w608 w630 w641 w651 w681 w697 w708 w723 w734 w746 w758 w769 w777 w794 w805 w817 w831 w844 w857 w870 w882 w887 w895 w901 w907 w915 w925 w936 w949 w963 w973 w980 w985 w993 w996 w1002 w1018 w1024 w1037 w1045 w1055 w1067 w1080 w1094 w1108 w1121 w1132 w1143 w1149 w1168 w1170 w1188 w1200 w1213 w1232] -> w492
          tunnel: [_ _ w502 w521 w533 w544 w559 w568 w580 w594 w600 w615 w629 w644 w652 w688 w698 w711 w722 w735 _ w757 w770 w781 w792 w804 w816 w830 w845 w856 w871 w883 w889 w894 w902 w908 w916 w926 w935 w948 w962 w972 w981 w986 w992 w997 w1003 w1017 w1025 w1036 w1046 w1054 w1066 w1079 w1093 w1109 w1122 _ w1139 w1148 w1164 w1171 w1184 w1196 w1211 w1231] -> w493
          tunnel: w491 -> [_ _ _ w507 w527 w542 w555 _ _ _ _ w617 w633 w645 w656 w684 w701 w716 w728 w737 w748 w760 w772 w786 w797 w809 w822 w833 w850 w862 w877 _ _ _ _ _ w921 _ w939 w944 w959 w977 _ _ _ _ w1008 w1021 _ w1040 _ w1059 w1071 w1085 w1099 _ _ _ _ _ _ w1177 _ _ _ w1235]
          tunnel: [_ "Unlock? (True)" _ _ _ _ _ _ _ _ _ _ _ _ _ _ _ _ _ _ _ _ _ _ _ _ _ _ _ _ _ _ _ _ _ _ _ _ _ _ _ _ _ _ _ _ _ _ _ _ _ _ _ _ _ _ _ _ _ _ _ _ _ _ _ _] -> w489
          event Timeout {
            n187 = event-data() -> ()  [unwired: 2 out]
          }
          event "stop": Value Change {
            n188 = event-data() -> ("NewVal"=w501:bool)  [unwired: 1 out]
          }
          event "Reset 4": Value Change {
            n189 = event-data() -> ()  [unwired: 2 out]
            n190 = call "CH_LM Error Clear.vi"("Meter Index"=w506, "error in (no error)"=errorcluster {"status"=FALSE, "code"=0, "source"=""} ("error out"), "Timeout / ms (3000)"=w503, "Lock Timeout / ms (1000)"=w503) -> ("Lock timed out"=w502:bool, "error out"=w504:errorcluster)  [unwired: 14 out]
          }
          event "AC Auto Off (On)", "AC Auto Off Timer (1 min)", "Battery Auto Off (On)", "Battery Auto Off Timer (1 min)", "State (On)": Value Change {
            n191 = event-data() -> ()  [unwired: 2 out]
            n192 = call "CH_LM Config Backlight.vi"("Meter Index"=w526, "AC Auto Off (Off)"="AC Auto Off (On)", "AC Auto Off Timer (1 min)"="AC Auto Off Timer (1 min)", "Battery Auto Off (Off)"="Battery Auto Off (On)", "Battery Auto Off Timer (1 min)"="Battery Auto Off Timer (1 min)", "error in (no error)"=w525, "State (On)"="State (On)", "Timeout / ms (3000)"=w522, "Action (query)"=w507, "Lock Timeout / ms (1000)"=w522) -> ("Lock timed out"=w519:bool, "Meter Index"=w524:i32, "error out"=w523:errorcluster)  [unwired: 7 out]
            n193 = call "CH_LM Config Backlight.vi"("Meter Index"=w524, "error in (no error)"=w523, "Timeout / ms (3000)"=w522, "Lock Timeout / ms (1000)"=w522) -> ("Lock timed out"=w520:bool, "State"=w513:bool, "AC Auto Off"=w512:bool, "AC Auto Off Timer / min"=w511:i32, "Battery Auto Off"=w510:bool, "Battery Auto Off Timer / min"=w509:i32, "error out"=w508:errorcluster)  [unwired: 6 in, 3 out]
            n194 = local write "Battery Auto Off Timer (1 min)"(w509) -> ()
            n195 = local write "AC Auto Off Timer (1 min)"(w511) -> ()
            n196 = local write "Battery Auto Off (On)"(w510) -> ()
            n197 = local write "AC Auto Off (On)"(w512) -> ()
            n198 = local write "State (On)"(w513) -> ()
            n199 = Or(x=w520, y=w519) -> (x .or. y?=w521:bool)
          }
          event "set Measurement Mode": Value Change {
            n200 = event-data() -> ()  [unwired: 2 out]
            n201 = call "CH_LM Config Measurement Mode.vi"("Meter Index"=w540, "Mode"="Mode", "Unit"="Unit", "error in (no error)"=w539, "Timeout / ms (3000)"=w534, "Action (query)"=w527, "Lock Timeout / ms (1000)"=w534) -> ("Lock timed out"=w531:bool, "Meter Index"=w538:i32, "error out"=w537:errorcluster)  [unwired: 10 out]
            n202 = call "CH_LM Config Measurement Mode.vi"("Meter Index"=w538, "error in (no error)"=w537, "Timeout / ms (3000)"=w534, "Lock Timeout / ms (1000)"=w534) -> ("Lock timed out"=w532:bool, "Mode"=w529:T12, "Unit"=w528:T11, "error out"=w530:errorcluster)  [unwired: 3 in, 9 out]
            n203 = local write "Mode"(w529) -> ()
            n204 = local write "Unit"(w528) -> ()
            n205 = Or(x=w532, y=w531) -> (x .or. y?=w533:bool)
          }
          event "set Wavelength": Value Change {
            n206 = event-data() -> ()  [unwired: 2 out]
            n207 = call "CH_LM Config Wavelength.vi"("Meter Index"=w553, "Wavelength / nm"="Wavelength / nm", "Option (Value)"="Option (Value)", "error in (no error)"=w552, "Timeout / ms (3000)"=w547, "Action (query)"=w542, "Lock Timeout / ms (1000)"=w547) -> ("Lock timed out"=w545:bool, "Meter Index"=w550:i32, "error out"=w549:errorcluster)  [unwired: 10 out]
            n208 = call "CH_LM Config Wavelength.vi"("Meter Index"=w550, "Option (Value)"="Option (Value)", "error in (no error)"=w549, "Timeout / ms (3000)"=w547, "Lock Timeout / ms (1000)"=w547) -> ("Lock timed out"=w546:bool, "Wavelength / nm"=w543:u32, "error out"=w548:errorcluster)  [unwired: 2 in, 10 out]
            n209 = local write "Wavelength / nm"(w543) -> ()
            n210 = Or(x=w546, y=w545) -> (x .or. y?=w544:bool)
          }
          event Value Change {
            n211 = event-data() -> ()  [unwired: 2 out]
            n212 = call "CH_LM Config Measurement Delivery Mode.vi"("Meter Index"=w564, "Delivery Mode"="Delivery Mode", "error in (no error)"=w563, "Timeout / ms (3000)"=w556, "Action (query)"=w555, "Lock Timeout / ms (1000)"=w556) -> ("Lock timed out"=w557:bool, "Meter Index"=w561:i32, "error out"=w562:errorcluster)  [unwired: 11 out]
            n213 = call "CH_LM Config Measurement Delivery Mode.vi"("Meter Index"=w561, "error in (no error)"=w562, "Timeout / ms (3000)"=w556, "Lock Timeout / ms (1000)"=w556) -> ("Lock timed out"=w558:bool, "Delivery Mode"=w560:T24, "error out"=w554:errorcluster)  [unwired: 2 in, 11 out]
            n214 = local write "Delivery Mode"(w560) -> ()
            n215 = Or(x=w558, y=w557) -> (x .or. y?=w559:bool)
          }
          event "Reset": Value Change {
            n216 = event-data() -> ()  [unwired: 2 out]
            n217 = call "Prompt for Calibration Password"() -> ("OK"=w566:bool)  [unwired: 2 in, 17 out]
            n218 = case shown="True" w566 {
              tunnel: w571 -> [_ w577]
              tunnel: w570 -> [w572 w576]
              tunnel: w569 -> [_ w575]
              tunnel: [_ w574] -> w568
              tunnel: [w572 w573] -> w567
              frame False {
              }
              frame True {
                n219 = call "CH_LM Reset.vi"("Meter Index"=w577, "error in (no error)"=w576, "Timeout / ms (3000)"=w575, "Lock Timeout / ms (1000)"=w575) -> ("Lock timed out"=w574:bool, "error out"=w573:errorcluster)  [unwired: 1 in, 13 out]
              }
            }
          }
          event "send SCPI": Value Change {
            n220 = event-data() -> ()  [unwired: 2 out]
            n221 = call "CH_LM Utility SCPI.vi"("Meter Index"=w583, "SCPI Command/Query"="SCPI Command/Query", "NofStrings (-1:all)"="NofStrings (-1:all)", "error in (no error)"=w582, "Timeout / ms (3000)"=w581, "Lock Timeout / ms (1000)"=w581) -> ("Lock timed out"=w580:bool, "Response"=→"Response":string, "Response Array"=→"Response Array":string[], "error out"=w579:errorcluster)  [unwired: 10 out]
          }
          event "Update Probe": Value Change {
            n222 = event-data() -> ()  [unwired: 2 out]
            n223 = call "CH_LM Utility Probe Information.vi"("Meter Index"=w598, "error in (no error)"=w597, "Timeout / ms (3000)"=w596, "Lock Timeout / ms (1000)"=w596) -> ("Model"=→"Probe Model":string, "Lock timed out"=w594:bool, "Probe Type"=→"Probe Type":T3, "Serial Number"=→"Serial Number":string, "Probe Qualifier"=→"Probe Qualifier":T2, "Calibration Date"=→"Calibration Date":timestamp, "Head Temperature"=→"Head Temperature":dbl[unit], "Responsitivity"=→"Responsitivity":dbl, "error out"=w595:errorcluster)  [unwired: 7 out]
          }
          event "Batch (start)": Value Change {
            n224 = event-data() -> ()  [unwired: 2 out]
            n225 = call "CH_LM Action Statistics StartStop.vi"("Meter Index"=w603, "Start/Stop (start)"="Batch (start)", "error in (no error)"=w602, "Timeout / ms (3000)"=w601, "Lock Timeout / ms (1000)"=w601) -> ("Lock timed out"=w600:bool, "error out"=w599:errorcluster)  [unwired: 13 out]
          }
          event "Time Stamp": Value Change {
            n226 = event-data() -> ()  [unwired: 2 out]
            n227 = call "CH_LM Utility Meter Information.vi"("Meter Index"=w619, "Date Format (MDY)"="Date Format (MDY)", "Time Stamp"="Time Stamp", "error in (no error)"=w618, "Timeout / ms (3000)"=w616, "Action (query)"=w617, "Lock Timeout / ms (1000)"=w616) -> ("Lock timed out"=w613:bool, "Meter Index"=w611:i32, "error out"=w612:errorcluster)  [unwired: 10 out]
            n228 = call "CH_LM Utility Meter Information.vi"("Meter Index"=w611, "error in (no error)"=w612, "Timeout / ms (3000)"=w616, "Lock Timeout / ms (1000)"=w616) -> ("Lock timed out"=w614:bool, "Meter Type"=→"Meter Type":T4, "Serial Number"=→"Serial Number":string, "Date Format"=w610:T13, "Time Stamp"=w609:timestamp, "Calibration Date"=→"Calibration Date":string, "error out"=w608:errorcluster)  [unwired: 3 in, 6 out]
            n229 = local write "Date Format (MDY)"(w610) -> ()
            n230 = local write "Time Stamp"(w609) -> ()
            n231 = Or(x=w614, y=w613) -> (x .or. y?=w615:bool)
          }
          event "Clear (false)", "Text (empty)", "Contrast (0.5)": Value Change {
            n232 = event-data() -> ()  [unwired: 2 out]
            n233 = call "CH_LM Config Display.vi"("Meter Index"=w635, "Contrast (0.5)"="Contrast (0.5)", "Text (empty)"="Text (empty)", "Clear (false)"="Clear (false)", "error in (no error)"=w634, "Timeout / ms (3000)"=w626, "Action (query)"=w633, "Lock Timeout / ms (1000)"=w626) -> ("Lock timed out"=w627:bool, "Meter Index"=w631:i32, "error out"=w632:errorcluster)  [unwired: 9 out]
            n234 = call "CH_LM Config Display.vi"("Meter Index"=w631, "error in (no error)"=w632, "Timeout / ms (3000)"=w626, "Lock Timeout / ms (1000)"=w626) -> ("Lock timed out"=w628:bool, "Contrast"=w624:dbl, "error out"=w630:errorcluster)  [unwired: 4 in, 9 out]
            n235 = local write "Contrast (0.5)"(w624) -> ()
            n236 = Or(x=w628, y=w627) -> (x .or. y?=w629:bool)
          }
          event Value Change {
            n237 = event-data() -> ()  [unwired: 2 out]
            n238 = call "CH_LM Config Analog Output Full Scale Voltage.vi"("Meter Index"=w647, "Analog Out \nFullscale Voltage (2V)"="Analog Out Fullscale Voltage (2V)", "error in (no error)"=w646, "Timeout / ms (3000)"=w636, "Action (query)"=w645, "Lock Timeout / ms (1000)"=w636) -> ("Lock timed out"=w639:bool, "Meter Index"=w643:i32, "error out"=w642:errorcluster)  [unwired: 1 in, 10 out]
            n239 = call "CH_LM Config Analog Output Full Scale Voltage.vi"("Meter Index"=w643, "error in (no error)"=w642, "Timeout / ms (3000)"=w636, "Lock Timeout / ms (1000)"=w636) -> ("Lock timed out"=w640:bool, "Analog Out \nFullscale Voltage"=w637:T8, "error out"=w641:errorcluster)  [unwired: 2 in, 11 out]
            n240 = local write "Analog Out Fullscale Voltage (2V)"(w637) -> ()
            n241 = Or(x=w640, y=w639) -> (x .or. y?=w644:bool)
          }
          event "Speedup Status": Value Change {
            w648 = 4
            n242 = event-data() -> ()  [unwired: 2 out]
            n243 = Cluster To Array(cluster="Speedup Status") -> (array=w660:bool[])
            n244 = for {
              N: w648 -> [_]
              tunnel: w663 -> [w680]
              tunnel: w661 -> [w674]
              tunnel: w660 -> [w677] mode=indexing
              shift-right: [w676] -> w658
              shift-left: w662 -> [w679]
              tunnel: [w675] -> w659
              tunnel: [w674] -> w657
              tunnel: w656 -> [w673]
              tunnel: [w672] -> w654 mode=indexing
              i -> [w678]
              n245 = call "CH_LM Config Speedup.vi"("Meter Index"=w680, "Speedup Mode (0)"=w678, "Status (On)"=w677, "error in (no error)"=w679, "Timeout / ms (3000)"=w674, "Action (query)"=w673, "Lock Timeout / ms (1000)"=w674) -> ("Lock timed out"=w672:bool, "Meter Index"=w675:i32, "error out"=w676:errorcluster)  [unwired: 10 out]
            }
            n246 = for {
              N: w648 -> [_]
              tunnel: w659 -> [w671]
              tunnel: w657 -> [w669]
              shift-right: [w667] -> w651
              shift-left: w658 -> [w670]
              tunnel: [w666] -> w655 mode=indexing
              tunnel: [w665] -> w650 mode=indexing
              i -> [w668]
              n247 = call "CH_LM Config Speedup.vi"("Meter Index"=w671, "Speedup Mode (0)"=w668, "error in (no error)"=w670, "Timeout / ms (3000)"=w669, "Lock Timeout / ms (1000)"=w669) -> ("Lock timed out"=w666:bool, "Status"=w665:bool, "error out"=w667:errorcluster)  [unwired: 2 in, 10 out]
            }
            n248 = Build Array (concatenate)(w655, w654) -> (w653:bool[])
            n249 = Or Array Elements(Boolean array=w653) -> (logical OR=w652:bool)
            n250 = Array To Cluster(array=w650) -> (cluster=w649:T29)
            n251 = local write "Speedup Status"(w649) -> ()
          }
          event Value Change {
            n252 = event-data() -> ()  [unwired: 2 out]
            n253 = local read "Probe Type"() -> (w683:T3)
            n254 = call "CH_LM Config Resolution.vi"("Meter Index"=w693, "Probe Type"=w683, "Resolution (3 1/2)"="Resolution (3 1/2)", "error in (no error)"=w692, "Timeout / ms (3000)"=w689, "Action (query)"=w684, "Lock Timeout / ms (1000)"=w689) -> ("Lock timed out"=w686:bool, "Meter Index"=w691:i32, "error out"=w690:errorcluster)  [unwired: 10 out]
            n255 = call "CH_LM Config Resolution.vi"("Meter Index"=w691, "Probe Type"=w683, "error in (no error)"=w690, "Timeout / ms (3000)"=w689, "Lock Timeout / ms (1000)"=w689) -> ("Lock timed out"=w687:bool, "Resolution (3 1/2)"=w682:T9, "error out"=w681:errorcluster)  [unwired: 2 in, 10 out]
            n256 = local write "Resolution (3 1/2)"(w682) -> ()
            n257 = Or(x=w687, y=w686) -> (x .or. y?=w688:bool)
          }
          event "WL correction (disable)": Value Change {
            n258 = event-data() -> ()  [unwired: 2 out]
            n259 = call "CH_LM Config Range Auto.vi"("Meter Index"=w705, "Auto Range (disable)"="WL correction (disable)", "error in (no error)"=w704, "Timeout / ms (3000)"=w699, "Action (query)"=w701, "Lock Timeout / ms (1000)"=w699) -> ("Lock timed out"=w695:bool, "Meter Index"=w703:i32, "error out"=w702:errorcluster)  [unwired: 11 out]
            n260 = call "CH_LM Config Range Auto.vi"("Meter Index"=w703, "error in (no error)"=w702, "Timeout / ms (3000)"=w699, "Lock Timeout / ms (1000)"=w699) -> ("Lock timed out"=w696:bool, "Auto Range"=w694:bool, "error out"=w697:errorcluster)  [unwired: 2 in, 11 out]
            n261 = local write "WL correction (disable)"(w694) -> ()
            n262 = Or(x=w696, y=w695) -> (x .or. y?=w698:bool)
          }
          event "set WL Table": Value Change {
            n263 = event-data() -> ()  [unwired: 2 out]
            n264 = call "CH_LM Config Wavelength Table Definition.vi"("Meter Index"=w718, "Wavelength Table"="Wavelength Table", "error in (no error)"=w717, "Timeout / ms (3000)"=w712, "Action (query)"=w716, "Lock Timeout / ms (1000)"=w712) -> ("Lock timed out"=w709:bool, "Meter Index"=w714:i32, "error out"=w713:errorcluster)  [unwired: 1 in, 10 out]
            n265 = call "CH_LM Config Wavelength Table Definition.vi"("Meter Index"=w714, "error in (no error)"=w713, "Timeout / ms (3000)"=w712, "Lock Timeout / ms (1000)"=w712) -> ("Lock timed out"=w710:bool, "Wavelength Table"=w707:u32[], "error out"=w708:errorcluster)  [unwired: 3 in, 10 out]
            n266 = local write "Wavelength Table"(w707) -> ()
            n267 = Array Size(array=w707) -> (size(s)=→"size":i32)
            n268 = Or(x=w710, y=w709) -> (x .or. y?=w711:bool)
          }
          event "Gain Compensation (disable)": Value Change {
            n269 = event-data() -> ()  [unwired: 2 out]
            n270 = call "CH_LM Config Gain Compensation State.vi"("Meter Index"=w730, "Gain Compensation (disable)"="Gain Compensation (disable)", "error in (no error)"=w729, "Timeout / ms (3000)"=w724, "Action (query)"=w728, "Lock Timeout / ms (1000)"=w724) -> ("Lock timed out"=w720:bool, "Meter Index"=w727:i32, "error out"=w726:errorcluster)  [unwired: 11 out]
            n271 = call "CH_LM Config Gain Compensation State.vi"("Meter Index"=w727, "error in (no error)"=w726, "Timeout / ms (3000)"=w724, "Lock Timeout / ms (1000)"=w724) -> ("Lock timed out"=w721:bool, "Gain Compensation"=w719:bool, "error out"=w723:errorcluster)  [unwired: 2 in, 11 out]
            n272 = local write "Gain Compensation (disable)"(w719) -> ()
            n273 = Or(x=w721, y=w720) -> (x .or. y?=w722:bool)
          }
          event "Compensation Factor (1.0)": Value Change {
            n274 = event-data() -> ()  [unwired: 2 out]
            n275 = call "CH_LM Config Gain Compensation.vi"("Meter Index"=w742, "Compensation Factor (1.0)"="Compensation Factor (1.0)", "error in (no error)"=w741, "Timeout / ms (3000)"=w736, "Action (query)"=w737, "Lock Timeout / ms (1000)"=w736) -> ("Lock timed out"=w732:bool, "Meter Index"=w739:i32, "error out"=w738:errorcluster)  [unwired: 11 out]
            n276 = call "CH_LM Config Gain Compensation.vi"("Meter Index"=w739, "error in (no error)"=w738, "Timeout / ms (3000)"=w736, "Lock Timeout / ms (1000)"=w736) -> ("Lock timed out"=w733:bool, "Compensation Factor"=w731:dbl, "error out"=w734:errorcluster)  [unwired: 2 in, 11 out]
            n277 = local write "Compensation Factor (1.0)"(w731) -> ()
            n278 = Or(x=w733, y=w732) -> (x .or. y?=w735:bool)
          }
          event "Area Correction (disable)": Value Change {
            n279 = event-data() -> ()  [unwired: 2 out]
            n280 = call "CH_LM Config Area Correction State.vi"("Meter Index"=w753, "Area Correction (disable)"="Area Correction (disable)", "error in (no error)"=w752, "Timeout / ms (3000)"=w747, "Action (query)"=w748, "Lock Timeout / ms (1000)"=w747) -> ("Lock timed out"=w744:bool, "Meter Index"=w751:i32, "error out"=w750:errorcluster)  [unwired: 11 out]
            n281 = call "CH_LM Config Area Correction State.vi"("Meter Index"=w751, "error in (no error)"=w750, "Timeout / ms (3000)"=w747, "Lock Timeout / ms (1000)"=w747) -> ("Lock timed out"=w745:bool, "Area Correction"=w743:bool, "error out"=w746:errorcluster)  [unwired: 2 in, 11 out]
            n282 = local write "Area Correction (disable)"(w743) -> ()
            n283 = Or(x=w745, y=w744) -> ()  [unwired: 1 out]
          }
          event "Aperture / cm² (1.0)": Value Change {
            n284 = event-data() -> ()  [unwired: 2 out]
            n285 = call "CH_LM Config Aperture.vi"("Meter Index"=w765, "Aperture / cm² (1.0)"="Aperture / cm² (1.0)", "error in (no error)"=w764, "Timeout / ms (3000)"=w759, "Action (query)"=w760, "Lock Timeout / ms (1000)"=w759) -> ("Lock timed out"=w755:bool, "Meter Index"=w762:i32, "error out"=w761:errorcluster)  [unwired: 11 out]
            n286 = call "CH_LM Config Aperture.vi"("Meter Index"=w762, "error in (no error)"=w761, "Timeout / ms (3000)"=w759, "Lock Timeout / ms (1000)"=w759) -> ("Lock timed out"=w756:bool, "Aperture / cm²"=w754:dbl, "error out"=w758:errorcluster)  [unwired: 2 in, 11 out]
            n287 = local write "Aperture / cm² (1.0)"(w754) -> ()
            n288 = Or(x=w756, y=w755) -> (x .or. y?=w757:bool)
          }
          event "Probe zero": Value Change {
            n289 = event-data() -> ()  [unwired: 2 out]
            n290 = call "CH_LM Action Probe Zero.vi"("Meter Index"=w776, "error in (no error)"=w775, "Timeout / ms (3000)"=w771, "Action (query)"=w772, "Lock Timeout / ms (1000)"=w771) -> ("Lock timed out"=w767:bool, "Meter Index"=w774:i32, "error out"=w773:errorcluster)  [unwired: 12 out]
            n291 = call "CH_LM Action Probe Zero.vi"("Meter Index"=w774, "error in (no error)"=w773, "Timeout / ms (3000)"=w771, "Lock Timeout / ms (1000)"=w771) -> ("Lock timed out"=w768:bool, "Zero Offset / W"=→"Zero Offset / W":dbl, "error out"=w769:errorcluster)  [unwired: 1 in, 12 out]
            n292 = Or(x=w768, y=w767) -> (x .or. y?=w770:bool)
          }
          event "Number of Pulses (0:Auto)": Value Change {
            n293 = event-data() -> ()  [unwired: 2 out]
            n294 = call "CH_LM Config Display Smoothing Size Pulse.vi"("Meter Index"=w788, "Number of Pulses (0:Auto)"="Number of Pulses (0:Auto)", "error in (no error)"=w787, "Timeout / ms (3000)"=w778, "Action (query)"=w786, "Lock Timeout / ms (1000)"=w778) -> ("Lock timed out"=w779:bool, "Meter Index"=w785:i32, "error out"=w784:errorcluster)  [unwired: 1 in, 10 out]
            n295 = call "CH_LM Config Display Smoothing Size Pulse.vi"("Meter Index"=w785, "error in (no error)"=w784, "Timeout / ms (3000)"=w778, "Lock Timeout / ms (1000)"=w778) -> ("Lock timed out"=w780:bool, "Number of Pulses"=w782:i32, "error out"=w777:errorcluster)  [unwired: 2 in, 11 out]
            n296 = local write "Number of Pulses (0:Auto)"(w782) -> ()
            n297 = Or(x=w780, y=w779) -> (x .or. y?=w781:bool)
          }
          event "Time / s (0:Auto)": Value Change {
            n298 = event-data() -> ()  [unwired: 2 out]
            n299 = call "CH_LM Config Display Smoothing Size Time.vi"("Meter Index"=w800, "Time / s (0:Auto)"="Time / s (0:Auto)", "error in (no error)"=w799, "Timeout / ms (3000)"=w793, "Action (query)"=w797, "Lock Timeout / ms (1000)"=w793) -> ("Lock timed out"=w790:bool, "Meter Index"=w796:i32, "error out"=w795:errorcluster)  [unwired: 1 in, 10 out]
            n300 = call "CH_LM Config Display Smoothing Size Time.vi"("Meter Index"=w796, "error in (no error)"=w795, "Timeout / ms (3000)"=w793, "Lock Timeout / ms (1000)"=w793) -> ("Lock timed out"=w791:bool, "Time / s"=w789:i32, "error out"=w794:errorcluster)  [unwired: 3 in, 10 out]
            n301 = local write "Time / s (0:Auto)"(w789) -> ()
            n302 = Or(x=w791, y=w790) -> (x .or. y?=w792:bool)
          }
          event "Restart Mode (f:manual)": Value Change {
            n303 = event-data() -> ()  [unwired: 2 out]
            n304 = call "CH_LM Config Statistics Restart Mode.vi"("Meter Index"=w812, "Restart Mode (f:manual)"="Restart Mode (f:manual)", "error in (no error)"=w811, "Timeout / ms (3000)"=w806, "Action (query)"=w809, "Lock Timeout / ms (1000)"=w806) -> ("Lock timed out"=w802:bool, "Meter Index"=w808:i32, "error out"=w807:errorcluster)  [unwired: 11 out]
            n305 = call "CH_LM Config Statistics Restart Mode.vi"("Meter Index"=w808, "error in (no error)"=w807, "Timeout / ms (3000)"=w806, "Lock Timeout / ms (1000)"=w806) -> ("Lock timed out"=w803:bool, "Restart Mode"=w801:bool, "error out"=w805:errorcluster)  [unwired: 2 in, 11 out]
            n306 = local write "Restart Mode (f:manual)"(w801) -> ()
            n307 = Or(x=w803, y=w802) -> (x .or. y?=w804:bool)
          }
          event "Number of Bins (7)": Value Change {
            n308 = event-data() -> ()  [unwired: 2 out]
            n309 = call "CH_LM Config Statistics Histogram Bin Count.vi"("Meter Index"=w824, "Number of Bins (7)"="Number of Bins (7)", "error in (no error)"=w823, "Timeout / ms (3000)"=w818, "Action (query)"=w822, "Lock Timeout / ms (1000)"=w818) -> ("Lock timed out"=w814:bool, "Meter Index"=w820:i32, "error out"=w819:errorcluster)  [unwired: 11 out]
            n310 = call "CH_LM Config Statistics Histogram Bin Count.vi"("Meter Index"=w820, "error in (no error)"=w819, "Timeout / ms (3000)"=w818, "Lock Timeout / ms (1000)"=w818) -> ("Lock timed out"=w815:bool, "Number of Bins"=w813:i32, "error out"=w817:errorcluster)  [unwired: 2 in, 11 out]
            n311 = local write "Number of Bins (7)"(w813) -> ()
            n312 = Or(x=w815, y=w814) -> (x .or. y?=w816:bool)
          }
          event "Batch Size (2)", "Sample Rate (1)": Value Change {
            n313 = event-data() -> ()  [unwired: 2 out]
            n314 = call "CH_LM Config Statistics Batch Size.vi"("Meter Index"=w838, "Batch Size (2)"="Batch Size (2)", "Sample Rate (1)"="Sample Rate (1)", "error in (no error)"=w837, "Timeout / ms (3000)"=w832, "Action (query)"=w833, "Lock Timeout / ms (1000)"=w832) -> ("Lock timed out"=w828:bool, "Meter Index"=w835:i32, "error out"=w834:errorcluster)  [unwired: 10 out]
            n315 = call "CH_LM Config Statistics Batch Size.vi"("Meter Index"=w835, "error in (no error)"=w834, "Timeout / ms (3000)"=w832, "Lock Timeout / ms (1000)"=w832) -> ("Lock timed out"=w829:bool, "Batch Size"=w827:i32, "Sample Rate"=w825:i32, "error out"=w831:errorcluster)  [unwired: 3 in, 9 out]
            n316 = local write "Sample Rate (1)"(w825) -> ()
            n317 = local write "Batch Size (2)"(w827) -> ()
            n318 = Or(x=w829, y=w828) -> (x .or. y?=w830:bool)
          }
          event "Sample Rate /Hz (10Hz)": Value Change {
            n319 = event-data() -> ()  [unwired: 2 out]
            n320 = call "CH_LM Config Statistics Batch Time.vi"("Meter Index"=w852, "Batch Time (00:01:00)"="Batch Time (00:01:00)", "Sample Rate /Hz (10Hz)"="Sample Rate /Hz (10Hz)", "error in (no error)"=w851, "Timeout / ms (3000)"=w846, "Action (query)"=w850, "Lock Timeout / ms (1000)"=w846) -> ("Lock timed out"=w842:bool, "Meter Index"=w848:i32, "error out"=w847:errorcluster)  [unwired: 10 out]
            n321 = call "CH_LM Config Statistics Batch Time.vi"("Meter Index"=w848, "error in (no error)"=w847, "Timeout / ms (3000)"=w846, "Lock Timeout / ms (1000)"=w846) -> ("Lock timed out"=w843:bool, "Batch Time"=w841:T21, "Sample Rate / Hz"=w839:dbl, "error out"=w844:errorcluster)  [unwired: 3 in, 9 out]
            n322 = local write "Batch Time (00:01:00)"(w841) -> ()
            n323 = local write "Sample Rate /Hz (10Hz)"(w839) -> ()
            n324 = Or(x=w843, y=w842) -> (x .or. y?=w845:bool)
          }
          event "Display Item List": Value Change {
            n325 = event-data() -> ()  [unwired: 2 out]
            n326 = call "CH_LM Config Statistics Display Item.vi"("Meter Index"=w864, "Display Item List"="Display Item List", "error in (no error)"=w863, "Timeout / ms (3000)"=w858, "Action (query)"=w862, "Lock Timeout / ms (1000)"=w858) -> ("Lock timed out"=w854:bool, "Meter Index"=w860:i32, "error out"=w859:errorcluster)  [unwired: 11 out]
            n327 = call "CH_LM Config Statistics Display Item.vi"("Meter Index"=w860, "error in (no error)"=w859, "Timeout / ms (3000)"=w858, "Lock Timeout / ms (1000)"=w858) -> ("Lock timed out"=w855:bool, "Display Item List"=w853:T20[], "error out"=w857:errorcluster)  [unwired: 2 in, 11 out]
            n328 = local write "Display Item List"(w853) -> ()
            n329 = Or(x=w855, y=w854) -> (x .or. y?=w856:bool)
          }
          event "Set Display Mode": Value Change {
            n330 = event-data() -> ()  [unwired: 2 out]
            n331 = local read "Display Mode"() -> (w865:T17)
            n332 = call "CH_LM Config Display Mode.vi"("Meter Index"=w879, "Display Mode"=w865, "Display Submode"="Display Submode", "View Mode"="View Mode", "error in (no error)"=w878, "Timeout / ms (3000)"=w872, "Action (query)"=w877, "Lock Timeout / ms (1000)"=w872) -> ("Lock timed out"=w868:bool, "Meter Index"=w874:i32, "error out"=w873:errorcluster)  [unwired: 9 out]
            n333 = call "CH_LM Config Display Mode.vi"("Meter Index"=w874, "Display Mode"=w865, "error in (no error)"=w873, "Timeout / ms (3000)"=w872, "Lock Timeout / ms (1000)"=w872) -> ("Lock timed out"=w869:bool, "Display Submode"=w867:T16, "View Mode"=w866:T15, "error out"=w870:errorcluster)  [unwired: 3 in, 8 out]
            n334 = local write "Display Submode"(w867) -> ()
            n335 = local write "View Mode"(w866) -> ()
            n336 = Or(x=w869, y=w868) -> (x .or. y?=w871:bool)
          }
          event "Update Catalog": Value Change {
            n337 = event-data() -> ()  [unwired: 2 out]
            n338 = call "CH_LM Action Configuration Catalog.vi"("Meter Index"=w886, "error in (no error)"=w885, "Timeout / ms (3000)"=w884, "Lock Timeout / ms (1000)"=w884) -> ("Lock timed out"=w883:bool, "Configuration Catalog"=w881:string[], "error out"=w882:errorcluster)  [unwired: 13 out]
            "Configuration Catalog" <- w881
            n339 = Array Size(array=w881) -> (size(s)=→"Number of files":i32)
          }
          event "Recall": Value Change {
            n340 = event-data() -> ()  [unwired: 2 out]
            n341 = call "CH_LM Action Configuration Recall.vi"("Meter Index"=w892, "Configuration File Name (\"\")"="Source File Name (\"\")", "error in (no error)"=w891, "Timeout / ms (3000)"=w890, "Lock Timeout / ms (1000)"=w890) -> ("Lock timed out"=w889:bool, "error out"=w887:errorcluster)  [unwired: 13 out]
          }
          event "Save": Value Change {
            n342 = event-data() -> ()  [unwired: 2 out]
            n343 = call "CH_LM Action Configuration Save.vi"("Meter Index"=w898, "Configuration File Name (\"\")"="Destination File Name (\"\")", "error in (no error)"=w897, "Timeout / ms (3000)"=w896, "Lock Timeout / ms (1000)"=w896) -> ("Lock timed out"=w894:bool, "error out"=w895:errorcluster)  [unwired: 13 out]
          }
          event "Rename": Value Change {
            n344 = event-data() -> ()  [unwired: 2 out]
            n345 = local read "Destination File Name (\"\")"() -> (w899:string)
            n346 = local read "Source File Name (\"\")"() -> (w900:string)
            n347 = call "CH_LM Action Configuration Rename.vi"("Meter Index"=w905, "Source File Name (\"\")"=w900, "Destination File Name (\"\")"=w899, "error in (no error)"=w904, "Timeout / ms (3000)"=w903, "Lock Timeout / ms (1000)"=w903) -> ("Lock timed out"=w902:bool, "error out"=w901:errorcluster)  [unwired: 12 out]
          }
          event "Delete": Value Change {
            n348 = event-data() -> ()  [unwired: 2 out]
            n349 = local read "Source File Name (\"\")"() -> (w906:string)
            n350 = call "CH_LM Action Configuration Delete.vi"("Meter Index"=w911, "Configuration File Name (\"\")"=w906, "error in (no error)"=w910, "Timeout / ms (3000)"=w909, "Lock Timeout / ms (1000)"=w909) -> ("Lock timed out"=w908:bool, "error out"=w907:errorcluster)  [unwired: 13 out]
          }
          event Value Change {
            n351 = event-data() -> ()  [unwired: 2 out]
            n352 = call "CH_LM Config Position Stability Cycle Duration.vi"("Meter Index"=w923, "Cycle Time (00:01:00)"="Cycle Time (00:01:00)", "error in (no error)"=w922, "Timeout / ms (3000)"=w917, "Action (query)"=w921, "Lock Timeout / ms (1000)"=w917) -> ("Lock timed out"=w913:bool, "Meter Index"=w919:i32, "error out"=w918:errorcluster)  [unwired: 11 out]
            n353 = call "CH_LM Config Position Stability Cycle Duration.vi"("Meter Index"=w919, "error in (no error)"=w918, "Timeout / ms (3000)"=w917, "Lock Timeout / ms (1000)"=w917) -> ("Lock timed out"=w914:bool, "Cycle Time"=w912:T21, "error out"=w915:errorcluster)  [unwired: 2 in, 11 out]
            n354 = local write "Cycle Time (00:01:00)"(w912) -> ()
            n355 = Or(x=w914, y=w913) -> (x .or. y?=w916:bool)
          }
          event "Start/Stop (start)": Value Change {
            n356 = event-data() -> ()  [unwired: 2 out]
            n357 = call "CH_LM Action Position Stability Cycle StartStop.vi"("Meter Index"=w929, "Start/Stop (start)"="Start/Stop (start)", "error in (no error)"=w928, "Timeout / ms (3000)"=w927, "Lock Timeout / ms (1000)"=w927) -> ("Lock timed out"=w926:bool, "error out"=w925:errorcluster)  [unwired: 13 out]
          }
          event Value Change {
            n358 = event-data() -> ()  [unwired: 2 out]
            n359 = call "CH_LM Config Trigger Source.vi"("Meter Index"=w941, "Trigger Source"="Trigger Source", "error in (no error)"=w940, "Timeout / ms (3000)"=w932, "Action (query)"=w939, "Lock Timeout / ms (1000)"=w932) -> ("Lock timed out"=w933:bool, "Meter Index"=w938:i32, "error out"=w937:errorcluster)  [unwired: 11 out]
            n360 = call "CH_LM Config Trigger Source.vi"("Meter Index"=w938, "error in (no error)"=w937, "Timeout / ms (3000)"=w932, "Lock Timeout / ms (1000)"=w932) -> ("Lock timed out"=w934:bool, "Trigger Source"=w930:T18, "error out"=w936:errorcluster)  [unwired: 2 in, 11 out]
            n361 = local write "Trigger Source"(w930) -> ()
            n362 = Or(x=w934, y=w933) -> (x .or. y?=w935:bool)
          }
          event "Trigger Level (5%)": Value Change {
            n363 = event-data() -> ()  [unwired: 2 out]
            n364 = call "CH_LM Config Trigger Level.vi"("Meter Index"=w953, "Trigger Level (5%)"="Trigger Level (5%)", "error in (no error)"=w952, "Timeout / ms (3000)"=w945, "Action (query)"=w944, "Lock Timeout / ms (1000)"=w945) -> ("Lock timed out"=w946:bool, "Meter Index"=w951:i32, "error out"=w950:errorcluster)  [unwired: 11 out]
            n365 = call "CH_LM Config Trigger Level.vi"("Meter Index"=w951, "error in (no error)"=w950, "Timeout / ms (3000)"=w945, "Lock Timeout / ms (1000)"=w945) -> ("Lock timed out"=w947:bool, "Trigger Level / %"=w942:dbl, "error out"=w949:errorcluster)  [unwired: 2 in, 11 out]
            n366 = local write "Trigger Level (5%)"(w942) -> ()
            n367 = Or(x=w947, y=w946) -> (x .or. y?=w948:bool)
          }
          event "Trigger Slope (pos.)", "Trigger Delay (0µs)": Value Change {
            n368 = event-data() -> ()  [unwired: 2 out]
            n369 = call "CH_LM Config Trigger External.vi"("Meter Index"=w967, "Trigger Slope (pos.)"="Trigger Slope (pos.)", "Trigger Delay (0µs)"="Trigger Delay (0µs)", "error in (no error)"=w966, "Timeout / ms (3000)"=w958, "Action (query)"=w959, "Lock Timeout / ms (1000)"=w958) -> ("Lock timed out"=w960:bool, "Meter Index"=w965:i32, "error out"=w964:errorcluster)  [unwired: 10 out]
            n370 = call "CH_LM Config Trigger External.vi"("Meter Index"=w965, "error in (no error)"=w964, "Timeout / ms (3000)"=w958, "Lock Timeout / ms (1000)"=w958) -> ("Lock timed out"=w961:bool, "Trigger Slope"=w955:bool, "Trigger Delay / µs"=w954:dbl, "error out"=w963:errorcluster)  [unwired: 3 in, 9 out]
            n371 = local write "Trigger Slope (pos.)"(w955) -> ()
            n372 = local write "Trigger Delay (0µs)"(w954) -> ()
            n373 = Or(x=w961, y=w960) -> (x .or. y?=w962:bool)
          }
          event Value Change {
            n374 = event-data() -> ()  [unwired: 2 out]
            n375 = call "CH_LM Config Trigger Bus Control.vi"("Meter Index"=w979, "Trigger Bus Control (2)"="Trigger Bus Control (2)", "error in (no error)"=w978, "Timeout / ms (3000)"=w969, "Action (query)"=w977, "Lock Timeout / ms (1000)"=w969) -> ("Lock timed out"=w970:bool, "Meter Index"=w975:i32, "error out"=w974:errorcluster)  [unwired: 11 out]
            n376 = call "CH_LM Config Trigger Bus Control.vi"("Meter Index"=w975, "error in (no error)"=w974, "Timeout / ms (3000)"=w969, "Lock Timeout / ms (1000)"=w969) -> ("Lock timed out"=w971:bool, "Trigger Bus Control"=w968:T19, "error out"=w973:errorcluster)  [unwired: 2 in, 11 out]
            n377 = local write "Trigger Bus Control (2)"(w968) -> ()
            n378 = Or(x=w971, y=w970) -> (x .or. y?=w972:bool)
          }
          event "Hold": Value Change {
            n379 = event-data() -> ()  [unwired: 2 out]
            n380 = call "CH_LM Action Trigger Bus Hold.vi"("Meter Index"=w984, "error in (no error)"=w983, "Timeout / ms (3000)"=w982, "Lock Timeout / ms (1000)"=w982) -> ("Lock timed out"=w981:bool, "error out"=w980:errorcluster)  [unwired: 14 out]
          }
          event "Release": Value Change {
            n381 = event-data() -> ()  [unwired: 2 out]
            n382 = call "CH_LM Action Trigger Bus Release.vi"("Meter Index"=w989, "error in (no error)"=w988, "Timeout / ms (3000)"=w987, "Lock Timeout / ms (1000)"=w987) -> ("Lock timed out"=w986:bool, "error out"=w985:errorcluster)  [unwired: 14 out]
          }
          event "Sequence ID (0)": Value Change {
            n383 = event-data() -> ()  [unwired: 2 out]
            n384 = call "CH_LM Action Trigger Sequence ID.vi"("Meter Index"=w995, "Sequence ID (0)"="Sequence ID (0)", "error in (no error)"=w994, "Timeout / ms (3000)"=w991, "Lock Timeout / ms (1000)"=w991) -> ("Lock timed out"=w992:bool, "error out"=w993:errorcluster)  [unwired: 13 out]
          }
          event "Pyroelectric Autoset": Value Change {
            n385 = event-data() -> ()  [unwired: 2 out]
            n386 = call "CH_LM Action Pyroelectric Autoset.vi"("Meter Index"=w1000, "error in (no error)"=w999, "Timeout / ms (3000)"=w998, "Lock Timeout / ms (1000)"=w998) -> ("Lock timed out"=w997:bool, "error out"=w996:errorcluster)  [unwired: 14 out]
          }
          event "Auto Range (disable)": Value Change {
            n387 = event-data() -> ()  [unwired: 2 out]
            n388 = call "CH_LM Config Range Auto.vi"("Meter Index"=w1010, "Auto Range (disable)"="Auto Range (disable)", "error in (no error)"=w1009, "Timeout / ms (3000)"=w1004, "Action (query)"=w1008, "Lock Timeout / ms (1000)"=w1004) -> ("Meter Index"=w1006:i32, "error out"=w1005:errorcluster)  [unwired: 12 out]
            n389 = call "CH_LM Config Range Auto.vi"("Meter Index"=w1006, "error in (no error)"=w1005, "Timeout / ms (3000)"=w1004, "Lock Timeout / ms (1000)"=w1004) -> ("Lock timed out"=w1003:bool, "Auto Range"=w1001:bool, "error out"=w1002:errorcluster)  [unwired: 2 in, 11 out]
            n390 = local write "Auto Range (disable)"(w1001) -> ()
          }
          event "Range Option (Value)", "Range": Value Change {
            n391 = event-data() -> ()  [unwired: 2 out]
            n392 = call "CH_LM Config Range.vi"("Meter Index"=w1023, "Range"="Range", "Option (Value)"="Range Option (Value)", "error in (no error)"=w1022, "Timeout / ms (3000)"=w1014, "Action (query)"=w1021, "Lock Timeout / ms (1000)"=w1014) -> ("Lock timed out"=w1015:bool, "Meter Index"=w1020:i32, "error out"=w1019:errorcluster)  [unwired: 10 out]
            n393 = call "CH_LM Config Range.vi"("Meter Index"=w1020, "Option (Value)"="Range Option (Value)", "error in (no error)"=w1019, "Timeout / ms (3000)"=w1014, "Lock Timeout / ms (1000)"=w1014) -> ("Lock timed out"=w1016:bool, "Granted Full Scale Range"=w1012:dbl, "error out"=w1018:errorcluster)  [unwired: 2 in, 10 out]
            n394 = local write "Range"(w1012) -> ()
            n395 = Or(x=w1016, y=w1015) -> (x .or. y?=w1017:bool)
          }
          event "Tune Clear": Value Change {
            n396 = event-data() -> ()  [unwired: 2 out]
            n397 = call "CH_LM Action Tune Clear.vi"("Meter Index"=w1028, "error in (no error)"=w1027, "Timeout / ms (3000)"=w1026, "Lock Timeout / ms (1000)"=w1026) -> ("Lock timed out"=w1025:bool, "error out"=w1024:errorcluster)  [unwired: 14 out]
          }
          event "Display Mode", "Direction (horizontal)": Value Change {
            n398 = event-data() -> ()  [unwired: 2 out]
            n399 = call "CH_LM Config Tune Zoom.vi"("Meter Index"=w1042, "Display Mode"="Display Mode", "Direction (horizontal)"="Direction (horizontal)", "Zoom Mode (1)"="Factor (1)", "error in (no error)"=w1041, "Timeout / ms (3000)"=w1029, "Action (query)"=w1040, "Lock Timeout / ms (1000)"=w1029) -> ("Lock timed out"=w1034:bool, "Meter Index"=w1039:i32, "error out"=w1038:errorcluster)  [unwired: 9 out]
            n400 = call "CH_LM Config Tune Zoom.vi"("Meter Index"=w1039, "Display Mode"="Display Mode", "Direction (horizontal)"="Direction (horizontal)", "error in (no error)"=w1038, "Timeout / ms (3000)"=w1029, "Lock Timeout / ms (1000)"=w1029) -> ("Lock timed out"=w1035:bool, "Zoom Mode"=w1033:T14, "error out"=w1037:errorcluster)  [unwired: 2 in, 9 out]
            n401 = local write "Factor (1)"(w1033) -> ()
            n402 = Or(x=w1035, y=w1034) -> (x .or. y?=w1036:bool)
          }
          event "Trend Cycle (start)": Value Change {
            n403 = event-data() -> ()  [unwired: 2 out]
            n404 = call "CH_LM Action Trend StartStop.vi"("Meter Index"=w1049, "Start/Stop (start)"="Trend Cycle (start)", "File Name (\"\")"="File Name (\"\")", "error in (no error)"=w1048, "Timeout / ms (3000)"=w1047, "Lock Timeout / ms (1000)"=w1047) -> ("Lock timed out"=w1046:bool, "error out"=w1045:errorcluster)  [unwired: 12 out]
          }
          event Value Change {
            n405 = event-data() -> ()  [unwired: 2 out]
            n406 = call "CH_LM Config Trend Zoom.vi"("Meter Index"=w1061, "Zoom Mode (1)"="Trend Zoom (1)", "error in (no error)"=w1060, "Timeout / ms (3000)"=w1051, "Action (query)"=w1059, "Lock Timeout / ms (1000)"=w1051) -> ("Lock timed out"=w1052:bool, "Meter Index"=w1057:i32, "error out"=w1056:errorcluster)  [unwired: 11 out]
            n407 = call "CH_LM Config Trend Zoom.vi"("Meter Index"=w1057, "error in (no error)"=w1056, "Timeout / ms (3000)"=w1051, "Lock Timeout / ms (1000)"=w1051) -> ("Lock timed out"=w1053:bool, "Zoom Mode"=w1050:T14, "error out"=w1055:errorcluster)  [unwired: 2 in, 11 out]
            n408 = local write "Trend Zoom (1)"(w1050) -> ()
            n409 = Or(x=w1053, y=w1052) -> (x .or. y?=w1054:bool)
          }
          event "Trend Histogram Bins (7)": Value Change {
            n410 = event-data() -> ()  [unwired: 2 out]
            n411 = call "CH_LM Config Trend Histogram Bin Count.vi"("Meter Index"=w1073, "Number of Bins (7)"="Trend Histogram Bins (7)", "error in (no error)"=w1072, "Timeout / ms (3000)"=w1063, "Action (query)"=w1071, "Lock Timeout / ms (1000)"=w1063) -> ("Lock timed out"=w1064:bool, "Meter Index"=w1069:i32, "error out"=w1068:errorcluster)  [unwired: 11 out]
            n412 = call "CH_LM Config Trend Histogram Bin Count.vi"("Meter Index"=w1069, "error in (no error)"=w1068, "Timeout / ms (3000)"=w1063, "Lock Timeout / ms (1000)"=w1063) -> ("Lock timed out"=w1065:bool, "Number of Bins"=w1062:i32, "error out"=w1067:errorcluster)  [unwired: 2 in, 11 out]
            n413 = local write "Trend Histogram Bins (7)"(w1062) -> ()
            n414 = Or(x=w1065, y=w1064) -> (x .or. y?=w1066:bool)
          }
          event "Trend Size (2)", "Sampling Rate (1)": Value Change {
            n415 = event-data() -> ()  [unwired: 2 out]
            n416 = call "CH_LM Config Trend Size.vi"("Meter Index"=w1087, "Trend Size (2)"="Trend Size (2)", "Sampling Rate (1)"="Sampling Rate (1)", "error in (no error)"=w1086, "Timeout / ms (3000)"=w1076, "Action (query)"=w1085, "Lock Timeout / ms (1000)"=w1076) -> ("Lock timed out"=w1077:bool, "Meter Index"=w1082:i32, "error out"=w1081:errorcluster)  [unwired: 10 out]
            n417 = call "CH_LM Config Trend Size.vi"("Meter Index"=w1082, "error in (no error)"=w1081, "Timeout / ms (3000)"=w1076, "Lock Timeout / ms (1000)"=w1076) -> ("Lock timed out"=w1078:bool, "Trend Size"=w1075:i32, "Sampling Rate"=w1074:i32, "error out"=w1080:errorcluster)  [unwired: 3 in, 9 out]
            n418 = local write "Sampling Rate (1)"(w1074) -> ()
            n419 = local write "Trend Size (2)"(w1075) -> ()
            n420 = Or(x=w1078, y=w1077) -> (x .or. y?=w1079:bool)
          }
          event "Sample Rate /Hz (10Hz) 2": Value Change {
            n421 = event-data() -> ()  [unwired: 2 out]
            n422 = call "CH_LM Config Trend Time.vi"("Meter Index"=w1101, "Trend Time (00:01:00)"="Trend Time (00:01:00)", "Sample Rate /Hz (10Hz)"="Sample Rate /Hz (10Hz) 2", "error in (no error)"=w1100, "Timeout / ms (3000)"=w1088, "Action (query)"=w1099, "Lock Timeout / ms (1000)"=w1088) -> ("Lock timed out"=w1091:bool, "Meter Index"=w1096:i32, "error out"=w1095:errorcluster)  [unwired: 10 out]
            n423 = call "CH_LM Config Trend Time.vi"("Meter Index"=w1096, "error in (no error)"=w1095, "Timeout / ms (3000)"=w1088, "Lock Timeout / ms (1000)"=w1088) -> ("Lock timed out"=w1092:bool, "Trend Time"=w1090:T21, "Sample Rate / Hz"=w1089:dbl, "error out"=w1094:errorcluster)  [unwired: 3 in, 9 out]
            n424 = local write "Sample Rate /Hz (10Hz) 2"(w1089) -> ()
            n425 = local write "Trend Time (00:01:00)"(w1090) -> ()
            n426 = Or(x=w1092, y=w1091) -> (x .or. y?=w1093:bool)
          }
          event "Read Catalog": Value Change {
            w1105 = u32 0 ("Catalog index")
            n427 = event-data() -> ()  [unwired: 2 out]
            n428 = property on="Catalog index" class="DigNum (strict)"("Value"=w1105) -> ()  [unwired: 2 in, 2 out]
            n429 = call "CH_LM DFM Catalog.vi"("Meter Index"=w1112, "error in (no error)"=w1111, "Timeout / ms (3000)"=w1110, "Lock Timeout / ms (1000)"=w1110) -> ("Lock timed out"=w1109:bool, "Bytes in use"=→"Bytes in use":i32, "Bytes available"=→"Bytes available":i32, "Catalog"=w1103:T27[], "error out"=w1108:errorcluster)  [unwired: 11 out]
            "Catalog" <- w1103
            n430 = Index Array(array=w1103, index=w1105) -> (element=→"File":T27)
            n431 = Array Size(array=w1103) -> (size(s)=→"Catalog size":i32)
          }
          event "Delete File": Value Change {
            n432 = event-data() -> ()  [unwired: 2 out]
            n433 = local read "Current working directoy"() -> (w1115:string)
            n434 = local read "Catalog index"() -> (w1119:u32)
            n435 = property on="Catalog" class="Arr (strict)"() -> ("Value"=w1120:T33[])  [unwired: 2 in, 2 out]
            n436 = Index Array(array=w1120, index=w1119) -> (element=w1118:T33)
            n437 = Unbundle By Name(w1118) -> ("File name"=w1114:string)
            n438 = Concatenate Strings(w1115, "\\" ("element"), w1114) -> (w1113:string)
            n439 = call "CH_LM DFM Delete File.vi"("Meter Index"=w1125, "Type"="Type", "Directory or File Name (\"\")"=w1113, "error in (no error)"=w1124, "Timeout / ms (3000)"=w1123, "Lock Timeout / ms (1000)"=w1123) -> ("Lock timed out"=w1122:bool, "error out"=w1121:errorcluster)  [unwired: 12 out]
          }
          event "Catalog index": Value Change {
            n440 = event-data() -> ()  [unwired: 2 out]
            n441 = local read "Catalog size"() -> (w1126:i32)
            n442 = property on="Catalog" class="Arr (strict)"() -> ("Value"=w1133:T33[])  [unwired: 2 in, 2 out]
            n443 = Decrement(x=w1126) -> (x-1=w1127:i32)
            n444 = In Range and Coerce(upper limit=w1127, x="Catalog index", lower limit=u32 0) -> (coerced(x)=w1128:u32)  [unwired: 1 out]
            n445 = property on="Catalog index" class="DigNum (strict)"("Value"=w1128) -> ()  [unwired: 2 in, 2 out]
            n446 = Index Array(array=w1133, index=w1128) -> (element=w1131:T33)
            n447 = property on="File" class="Clust (strict)"("Value"=w1131) -> ()  [unwired: 2 in, 2 out]
          }
          event "Rename": Value Change {
            n448 = event-data() -> ()  [unwired: 2 out]
            n449 = local read "Current working directoy"() -> (w1136:string)
            n450 = local read "Catalog index"() -> (w1145:u32)
            n451 = property on="Catalog" class="Arr (strict)"() -> ("Value"=w1146:T33[])  [unwired: 2 in, 2 out]
            n452 = Index Array(array=w1146, index=w1145) -> (element=w1144:T33)
            n453 = Unbundle By Name(w1144) -> ("File name"=w1135:string)
            n454 = Concatenate Strings(w1136, "\\" ("element"), w1135) -> (w1134:string)
            n455 = call "CH_LM DFM Rename.vi"("Meter Index"=w1142, "Source Name (\"\")"=w1134, "Destination Name (\"\")"="Destination Name (\"\")", "error in (no error)"=w1141, "Timeout / ms (3000)"=w1140, "Lock Timeout / ms (1000)"=w1140) -> ("Lock timed out"=w1139:bool, "error out"=w1143:errorcluster)  [unwired: 12 out]
          }
          event "Copy File": Value Change {
            n456 = event-data() -> ()  [unwired: 2 out]
            n457 = local read "Destination Name (\"\")"() -> (w1151:string)
            n458 = local read "Catalog index"() -> (w1158:u32)
            n459 = property on="Catalog" class="Arr (strict)"() -> ("Value"=w1159:T33[])  [unwired: 2 in, 2 out]
            n460 = Index Array(array=w1159, index=w1158) -> (element=w1157:T33)
            n461 = local read "Current working directoy"() -> (w1155:string)
            n462 = Unbundle By Name(w1157) -> ("File name"=w1154:string)
            n463 = Concatenate Strings(w1155, "\\" ("element"), w1154) -> (w1152:string)
            n464 = call "CH_LM DFM Copy File.vi"("Meter Index"=w1153, "Source Name (\"\")"=w1152, "Destination Name (\"\")"=w1151, "error in (no error)"=w1150, "Timeout / ms (3000)"=w1147, "Lock Timeout / ms (1000)"=w1147) -> ("Lock timed out"=w1148:bool, "error out"=w1149:errorcluster)  [unwired: 12 out]
          }
          event "Create Directory": Value Change {
            n465 = local read "Current working directoy"() -> (w1163:string)
            n466 = event-data() -> ()  [unwired: 2 out]
            n467 = local read "Destination Name (\"\")"() -> (w1161:string)
            n468 = Concatenate Strings(w1163, "\\" ("element"), w1161) -> (w1160:string)
            n469 = call "CH_LM DFM Create Directory.vi"("Meter Index"=w1167, "Directory Name (\"\")"=w1160, "error in (no error)"=w1166, "Timeout / ms (3000)"=w1165, "Lock Timeout / ms (1000)"=w1165) -> ("Lock timed out"=w1164:bool, "error out"=w1168:errorcluster)  [unwired: 13 out]
          }
          event "Change Directory": Value Change {
            n470 = event-data() -> ()  [unwired: 2 out]
            n471 = local read "Destination Name (\"\")"() -> (w1178:string)
            n472 = call "CH_LM DFM Change Directory.vi"("Meter Index"=w1180, "Directory Name (\"\")"=w1178, "error in (no error)"=w1179, "Timeout / ms (3000)"=w1174, "Action (query)"=w1177, "Lock Timeout / ms (1000)"=w1174) -> ("Lock timed out"=w1172:bool, "Meter Index"=w1176:i32, "error out"=w1175:errorcluster)  [unwired: 11 out]
            n473 = call "CH_LM DFM Change Directory.vi"("Meter Index"=w1176, "error in (no error)"=w1175, "Timeout / ms (3000)"=w1174, "Lock Timeout / ms (1000)"=w1174) -> ("Lock timed out"=w1173:bool, "Woring Directory"=→"Current working directoy":string, "error out"=w1170:errorcluster)  [unwired: 2 in, 11 out]
            n474 = Or(x=w1173, y=w1172) -> (x .or. y?=w1171:bool)
          }
          event "Store into File": Value Change {
            n475 = event-data() -> ()  [unwired: 2 out]
            n476 = local read "Current working directoy"() -> (w1182:string)
            n477 = local read "Destination Name (\"\")"() -> (w1181:string)
            n478 = Concatenate Strings(w1182, "\\" ("element"), w1181) -> ()  [unwired: 1 out]
            n479 = call "CH_LM DFM Store File.vi"("Meter Index"=w1187, "File Name (\"\")"=w1181, "error in (no error)"=w1186, "Timeout / ms (3000)"=w1185, "Lock Timeout / ms (1000)"=w1185) -> ("Lock timed out"=w1184:bool, "error out"=w1188:errorcluster)  [unwired: 13 out]
          }
          event "Load from File": Value Change {
            n480 = event-data() -> ()  [unwired: 2 out]
            n481 = local read "Current working directoy"() -> (w1194:string)
            n482 = local read "Catalog index"() -> (w1191:u32)
            n483 = property on="Catalog" class="Arr (strict)"() -> ("Value"=w1192:T33[])  [unwired: 2 in, 2 out]
            n484 = Index Array(array=w1192, index=w1191) -> (element=w1190:T33)
            n485 = Unbundle By Name(w1190) -> ("File name"=w1189:string)
            n486 = Concatenate Strings(w1194, "\\" ("element"), w1189) -> (w1193:string)
            n487 = call "CH_LM DFM Load File.vi"("Meter Index"=w1199, "File Name (\"\")"=w1193, "error in (no error)"=w1198, "Timeout / ms (3000)"=w1197, "Lock Timeout / ms (1000)"=w1197) -> ("Lock timed out"=w1196:bool, "error out"=w1200:errorcluster)  [unwired: 13 out]
          }
          event "Download": Value Change {
            n488 = event-data() -> ()  [unwired: 2 out]
            n489 = local read "Current working directoy"() -> (w1203:string)
            n490 = local read "Catalog index"() -> (w1209:u32)
            n491 = property on="Catalog" class="Arr (strict)"() -> ("Value"=w1210:T33[])  [unwired: 2 in, 2 out]
            n492 = Index Array(array=w1210, index=w1209) -> (element=w1208:T33)
            n493 = Unbundle By Name(w1208) -> ("File name"=w1202:string)
            n494 = Concatenate Strings(w1203, "\\" ("element"), w1202) -> (w1201:string)
            n495 = Empty String/Path?(string/path="Destination (empty path)") -> (empty?=w1207:bool)
            n496 = case shown="False" w1207 {
              tunnel: w1215 -> [w1222 _]
              tunnel: w1214 -> [w1221 w1224]
              tunnel: [w1220 w1224] -> w1213
              tunnel: w1212 -> [w1219 _]
              tunnel: [w1218 _] -> w1211
              tunnel: w1201 -> [w1217 _]
              tunnel: "Destination (empty path)" -> [w1216 _]
              tunnel: "Please, select a filename first!" -> [_ w1223]
              frame False {
                n497 = call "CH_LM DFM Downoad File.vi"("Meter Index"=w1222, "File Name (\"\")"=w1217, "Destination (empty path)"=w1216, "error in (no error)"=w1221, "Timeout / ms (3000)"=w1219, "Lock Timeout / ms (1000)"=w1219) -> ("Lock timed out"=w1218:bool, "error out"=w1220:errorcluster)  [unwired: 12 out]
              }
              frame True {
                n498 = One Button Dialog(message=w1223) -> ()  [unwired: 2 out]
              }
            }
          }
          event "Header (disable)", "Data Tokens": Value Change {
            n499 = event-data() -> ()  [unwired: 2 out]
            n500 = call "CH_LM Config Data Header.vi"("Meter Index"=w1238, "Data Header (disable)"="Header (disable)", "Data Tokens"="Data Tokens", "error in (no error)"=w1237, "Timeout / ms (3000)"=w1228, "Action (query)"=w1235, "Lock Timeout / ms (1000)"=w1228) -> ("Lock timed out"=w1229:bool, "Meter Index"=w1234:i32, "error out"=w1233:errorcluster)  [unwired: 10 out]
            n501 = call "CH_LM Config Data Header.vi"("Meter Index"=w1234, "error in (no error)"=w1233, "Timeout / ms (3000)"=w1228, "Lock Timeout / ms (1000)"=w1228) -> ("Lock timed out"=w1230:bool, "Data Header"=w1227:bool, "Data Tokens"=w1225:T25[], "error out"=w1232:errorcluster)  [unwired: 3 in, 9 out]
            n502 = local write "Header (disable)"(w1227) -> ()
            n503 = local write "Data Tokens"(w1225) -> ()
            n504 = Or(x=w1230, y=w1229) -> (x .or. y?=w1231:bool)
          }
        }
        "Lock timed out" <- w493
        "Event error" <- w492
        n505 = call <vilib>:"Simple Error Handler.vi"("error in (no error)"=w492) -> ()  [unwired: 1 in, 8 out]
        "GUI Loop" <- w490
      }
      "stopping" <- w65
      n506 = while "Polling Loop" {
        tunnel: w34 -> [w182]
        tunnel: [w178] -> w82
        tunnel: w27 -> [w177]
        shift-right: [w179] -> w62
        shift-left: w39 -> [w181]
        tunnel: errorcluster {"status"=FALSE, "code"=0, "source"=""} ("error in (no error)") -> [w183]
        tunnel: [w177] -> w72
        stop <- w180 stop-if-true
        n507 = case shown="True" "Polling active" {
          tunnel: w183 -> [_ w209]
          tunnel: w182 -> [w186 w208]
          tunnel: w181 -> [w185 w207]
          tunnel: [w185 w203] -> w179
          tunnel: [w186 w195] -> w178
          tunnel: w177 -> [_ w190]
          frame False {
            n508 = Wait Until Next ms Multiple(millisecond multiple=u32 250) -> ()  [unwired: 1 out]
          }
          frame True {
            n509 = call "CH_LM Utility System Status.vi"("Meter Index"=w208, "error in (no error)"=w207, "Timeout / ms (3000)"=w190, "Lock Timeout / ms (1000)"=w190) -> ("Lock timed out"=w205:bool, "Meter Index"=w193:i32, "System Status"=w200:T28, "Status Description"=→"Status Description":string, "error out"=w192:errorcluster)  [unwired: 11 out]
            n510 = Number To Boolean Array(number=w200) -> (Boolean array=w199:bool[])
            n511 = call "CH_LM Utility Probe Information.vi"("Meter Index"=w193, "error in (no error)"=w192, "Timeout / ms (3000)"=w190, "Lock Timeout / ms (1000)"=w190) -> ("Lock timed out"=w191:bool, "Meter Index"=w195:i32, "Head Temperature"=w196:dbl[unit], "error out"=w194:errorcluster)  [unwired: 12 out]
            n512 = Array Subset(array=w199, length=11) -> (w198:bool[])  [unwired: 1 in]
            n513 = local write "Head Temperature"(w196) -> ()
            n514 = Array To Cluster(array=w198) -> (cluster=→"Status":T30)
            n515 = Compound Arithmetic op=OR(w191, w205) -> (w204:bool)
            n516 = local write "Lock timed out"(w204) -> ()
            n517 = Select(t=w209, s="Reset 2", f=w194) -> (s? t:f=w203:errorcluster)
            "Polling error" <- w203
            n518 = Max & Min(x="Intervall / ms", y=u32 100) -> (max(x,y)=w188:u32)  [unwired: 1 out]
            n519 = Unbundle By Name(w203) -> ("status"=→"Polling error":bool)
            n520 = Wait Until Next ms Multiple(millisecond multiple=w188) -> ()  [unwired: 1 out]
          }
        }
        n521 = local read "stopping"() -> (w180:bool)
      }
      n522 = Select(t=w63, s=w63, f=w62) -> (s? t:f=w61:errorcluster)
      n523 = Select(t=w61, s=w61, f=w81) -> (s? t:f=w60:errorcluster)
      n524 = Select(t=w60, s=w60, f=w58) -> (s? t:f=w59:errorcluster)
      n525 = call "CH_LM Close.vi"("Meter Index"=w82, "Unlock? (True)"=w38, "error in (no error)"=w59, "Timeout / ms (3000)"=w72, "Lock Timeout / ms (1000)"=w72) -> ("error out"=w83:errorcluster)  [unwired: 14 out]
    }
    frame Error {
    }
  }
  n526 = local write "stopping"(w7) -> ()
  n527 = call <vilib>:"Simple Error Handler.vi"("error in (no error)"=w14) -> ()  [unwired: 1 in, 8 out]
